vi "dI-dV(V) at various H_MFLI_MF-MD_K3636B_measureR_PK_V4.0_withaveraging.vi"() -> ()   [LabVIEW 2016]
uses:
  <instrlib>/Zurich Instruments LabOne/Public/Data/ziTypeDemodSampleSingle.ctl
  <instrlib>/Keithley 2600 Series/Public/Configure/Source/Configure Source (Limit).vi
  <instrlib>/Keithley 2600 Series/Public/Configure/Source/Configure Source (Range).vi
  <instrlib>/Zurich Instruments LabOne/Public/Configure/ziSetValueDouble.vi
  <instrlib>/Zurich Instruments LabOne/Public/Configure/ziGetValueDemodSampleEx.vi
  <instrlib>/Zurich Instruments LabOne/Zurich Instruments LabOne.lvlib
  <instrlib>/Keithley 2600 Series/Keithley 2600 Series.lvlib
panel:
  in  "MFLI autorange":bool
  in  "MFLI averaging":i32=100
  in  "Resistance used for DC (ohm)":dbl=20000000.0 format="%#_13g"
  in  "DC Current Limit (A)":dbl=0.001 format="%#_13g"
  in  "Keithley 2636B (channelA)":refnum<visa-resource-name>="GPIB0::26::INSTR"
  in  "Field ramp rate (T/min)":string="0.05"
  in  "Step 2":dbl[](array[numeric])=[0.01] min=-3000.0 max=3000.0 format="%.1e"
  in  "To 2":dbl[](array[numeric])=[1.0] min=-3000.0 max=3000.0 format="%.1e"
  in  "From 2":dbl[](array[numeric])=[1.0] min=-3000.0 max=3000.0 format="%.1e"
  in  "Magnet IP Address":string="169.254.239.127"
  in  "Magnetic field stabilization time (s)":dbl=10.0 format="%#_13g"
  out "Magnetic Field (T)":dbl=-9.479e-06 format="%#_13g"
  in  "DC Voltage averaging":dbl=20.0 format="%#_13g"
  out "Demod Sample Out 2":T1={"Timestamps (ticks)"=130270697085950, "X (Vrms)"=2.9261878078642585e-10, "Y (Vrms)"=-9.326090743141773e-11, "Osc Phase (deg)"=2.705175119436328, "Freq (Hz)"=137.91900016713043, "DIO"=0, "AuxIn0 (V)"=-1.5994189965713304, "AuxIn1 (V)"=0.0, "Trigger"=768}
  out "Demod Sample Out":T1={"Timestamps (ticks)"=130270395958270, "X (Vrms)"=1.8633428954504745e-05, "Y (Vrms)"=-1.3912734080062926e-05, "Osc Phase (deg)"=1.8681968520462253, "Freq (Hz)"=137.91900016713043, "DIO"=0, "AuxIn0 (V)"=-1.599753673071973, "AuxIn1 (V)"=0.0003336581285111606, "Trigger"=768}
  out "Vset (V)":dbl=-1.5999999999999879
  in  "stop":bool
  out "Time(s)":dbl=17491.89
  in  "Delay (s)":dbl=6.0
  out "dI/dV (S)":dbl=1.3195690059568667e-05
  out "dV (V)":dbl=2.3236791935984393e-05
  out "dI (A)":dbl=3.066255043659346e-10
  in  "MFLI Address":string="DEV4382"
  out "DC Voltage (V)":dbl=0.0024357376114999994
  in  "Folder":path=path "D:/Pranava/Data/STS/MA2087"
  out "dI/dV vs DC Bias (V)":cluster{dbl, "Field Reading":dbl}[](graph)=[{-0.0016267571685000004, "Field Reading"=1.2499190504022442e-05}, {-0.0016293047665, "Field Reading"=1.343983352593105e-05}, {-0.0016220483485, "Field Reading"=1.3498901551089376e-05}, {-0.0016165598575000003, "Field Reading"=1.3388711055940132e-05}, {-0.001611980558, "Field Reading"=1.3461634755634268e-05}, {-0.0016065861309999998, "Field Reading"=1.341362700532847e-05}, {-0.001602110838, "Field Reading"=1.3469326656062633e-05}, {-0.001603791602, "Field Reading"=1.3450198778996813e-05}, {-0.0016051868515, "Field Reading"=1.3453781776488028e-05}, {-0.0015975631075, "Field Reading"=1.3419416925134238e-05}, {-0.0015943920469999998, "Field Reading"=1.3462487063099248e-05}, {-0.001587995701, "Field Reading"=1.3450573702072532e-05}, {-0.0015837433415, "Field Reading"=1.3428263446816707e-05}, {-0.0015828466714999999, "Field Reading"=1.3393928336058793e-05}, {-0.0015733770785, "Field Reading"=1.3409612424077186e-05}, {-0.0015723401285000001, "Field Reading"=1.3483281690764093e-05}, {-0.001573338908, "Field Reading"=1.3468924481084309e-05}, {-0.0015673728475, "Field Reading"=1.3484666473714511e-05}, {-0.0015648761185, "Field Reading"=1.3459017041334516e-05}, {-0.0015634323450000002, "Field Reading"=1.3444091577240615e-05}, {-0.0015604055610000003, "Field Reading"=1.346636342471481e-05}, {-0.0015566468755, "Field Reading"=1.3440322960534301e-05}, {-0.0015575937835, "Field Reading"=1.3469711736300209e-05}, {-0.001552576611, "Field Reading"=1.3488882189349033e-05}, {-0.0015498932484999998, "Field Reading"=1.353533220023797e-05}, {-0.00154556704, "Field Reading"=1.3484237808051385e-05}, {-0.0015367533970000002, "Field Reading"=1.3408673038652877e-05}, {-0.0015292438589999996, "Field Reading"=1.3347996439904072e-05}, {-0.0015202704415000002, "Field Reading"=1.3380685506463923e-05}, {-0.0015157290055000001, "Field Reading"=1.3353547371126122e-05}, {-0.001518163067, "Field Reading"=1.3343450621350141e-05}, {-0.001513959626, "Field Reading"=1.3409316825027622e-05}, {-0.0015079468985, "Field Reading"=1.3565802247876391e-05}, {-0.00150523147, "Field Reading"=1.3366072109737657e-05}, {-0.0015025157965, "Field Reading"=1.3503176669159866e-05}, {-0.0015006006585000001, "Field Reading"=1.3475950682446334e-05}, {-0.0014965097129999998, "Field Reading"=1.343269307655852e-05}, {-0.0014928501455, "Field Reading"=1.3481127330206819e-05}, {-0.0014863147765, "Field Reading"=1.349537528914492e-05}, {-0.0014858813695000001, "Field Reading"=1.3464024342252269e-05}, {-0.0014759853594999998, "Field Reading"=1.3532450573952814e-05}, {-0.0014792820840000003, "Field Reading"=1.3467630784037758e-05}, {-0.0014737221895000003, "Field Reading"=1.3493114600583547e-05}, {-0.0014732275255000002, "Field Reading"=1.341814309027668e-05}, {-0.0014720142794999998, "Field Reading"=1.3430107894144245e-05}, {-0.0014674228615000002, "Field Reading"=1.3458062901131014e-05}, {-0.0014639780044999999, "Field Reading"=1.337799175960371e-05}, {-0.0014586194074999999, "Field Reading"=1.3432931895040972e-05}, {-0.0014546810515000002, "Field Reading"=1.3377936281541803e-05}, {-0.0014555862725000002, "Field Reading"=1.3440225961101887e-05}, {-0.0014500533295, "Field Reading"=1.3316922206414297e-05}, {-0.0014419232575, "Field Reading"=1.333479852156618e-05}, {-0.001439833057, "Field Reading"=1.335961205669311e-05}, {-0.001438517271, "Field Reading"=1.3276100719086655e-05}, {-0.001434182186, "Field Reading"=1.3414999580139993e-05}, {-0.0014277051765000004, "Field Reading"=1.3313685209980852e-05}, {-0.00142267889, "Field Reading"=1.3448885663949112e-05}, {-0.0014155909575, "Field Reading"=1.339123183517665e-05}, {-0.0014156524565, "Field Reading"=1.3297227349395088e-05}, {-0.0014124035680000001, "Field Reading"=1.3293565095925792e-05}, {-0.0014109490645, "Field Reading"=1.3394356468614784e-05}, {-0.001402366442, "Field Reading"=1.3391601134549928e-05}, {-0.001403825126, "Field Reading"=1.3292560889770096e-05}, {-0.0013966000125000002, "Field Reading"=1.3271969364171561e-05}, {-0.001394491805, "Field Reading"=1.3266411947286085e-05}, {-0.0013886783535, "Field Reading"=1.3363185326936124e-05}, {-0.0013879851079999998, "Field Reading"=1.3296944610611628e-05}, {-0.0013861102605, "Field Reading"=1.3375920541979456e-05}, {-0.001376159754, "Field Reading"=1.3268301330598542e-05}, {-0.0013715085824999999, "Field Reading"=1.3152900070607564e-05}, {-0.0013698944995, "Field Reading"=1.314215168062357e-05}, {-0.001366914667, "Field Reading"=1.3243900076650863e-05}, {-0.0013582629245000003, "Field Reading"=1.3197203437224588e-05}, {-0.0013513427565, "Field Reading"=1.3298167481611889e-05}, {-0.001352901842, "Field Reading"=1.3191445816026105e-05}, {-0.0013482640735, "Field Reading"=1.3131854012322067e-05}, {-0.0013431525900000003, "Field Reading"=1.319622184301407e-05}, {-0.0013453806239999999, "Field Reading"=1.3236450043175786e-05}, {-0.001338256563, "Field Reading"=1.3067235288946016e-05}, {-0.0013330496975, "Field Reading"=1.3278259509809853e-05}, {-0.001334601536, "Field Reading"=1.3161782791668972e-05}, {-0.0013293076895000001, "Field Reading"=1.3153363931625601e-05}, {-0.001328445928, "Field Reading"=1.3266280146530614e-05}, {-0.001323545566, "Field Reading"=1.3230633385568305e-05}, {-0.0013212523805, "Field Reading"=1.3153530500532615e-05}, {-0.001313054419, "Field Reading"=1.306718664169635e-05}, {-0.00131050229, "Field Reading"=1.3035829727727256e-05}, {-0.0013093692279999999, "Field Reading"=1.301171160959137e-05}, {-0.001300491978, "Field Reading"=1.3025217563977052e-05}, {-0.001291491248, "Field Reading"=1.2927163061100772e-05}, {-0.0012919785895, "Field Reading"=1.2950635606816967e-05}, {-0.0012839753905000003, "Field Reading"=1.295778636070639e-05}, {-0.001286123235, "Field Reading"=1.3035587121306979e-05}, {-0.001282255743, "Field Reading"=1.29379216298443e-05}, {-0.0012749608365, "Field Reading"=1.291957727591729e-05}, {-0.0012758108629999999, "Field Reading"=1.282723994321026e-05}, {-0.0012722698105000001, "Field Reading"=1.2806403042037306e-05}, {-0.001265646766, "Field Reading"=1.2866015068675188e-05}, {-0.0012694931415, "Field Reading"=1.2843347976402634e-05}, {-0.0012635237225, "Field Reading"=1.2985607427098843e-05}, {-0.0012617351054999997, "Field Reading"=1.3006933428484992e-05}, {-0.0012597806045, "Field Reading"=1.2885230079994883e-05}, {-0.0012488438765, "Field Reading"=1.2793535568477117e-05}, {-0.001242964541, "Field Reading"=1.2779432928316403e-05}, {-0.0012412559555, "Field Reading"=1.275312692545066e-05}, {-0.001240000649, "Field Reading"=1.2823591948584074e-05}, {-0.0012338296425, "Field Reading"=1.2753142420891901e-05}, {-0.0012334313899999999, "Field Reading"=1.260784282033363e-05}, {-0.0012307593545000002, "Field Reading"=1.2678998567641228e-05}, {-0.0012226835155000001, "Field Reading"=1.2531960406984556e-05}, {-0.0012170625415000003, "Field Reading"=1.2534788440635036e-05}, {-0.001215300631, "Field Reading"=1.2713738859126119e-05}, {-0.001214893501, "Field Reading"=1.2578666495750338e-05}, {-0.0012074607665, "Field Reading"=1.2623503148142356e-05}, {-0.0012017656785, "Field Reading"=1.2643045434630556e-05}, {-0.0011959136775, "Field Reading"=1.2531358907979804e-05}, {-0.001192863882, "Field Reading"=1.2682876125580679e-05}, {-0.001185345928, "Field Reading"=1.250172466195837e-05}, {-0.0011869023915000003, "Field Reading"=1.2401388355506459e-05}, {-0.001178852282, "Field Reading"=1.2735540228021439e-05}, {-0.0011705313045, "Field Reading"=1.2529360874641979e-05}, {-0.0011713601725000002, "Field Reading"=1.2406007363184931e-05}, {-0.001167284147, "Field Reading"=1.2562327760527226e-05}, {-0.0011657835375, "Field Reading"=1.2423839516376826e-05}, {-0.0011559746239999998, "Field Reading"=1.2409473414314111e-05}, {-0.0011557333085, "Field Reading"=1.223456105451975e-05}, {-0.00115341717, "Field Reading"=1.2267935976857073e-05}, {-0.0011506243345, "Field Reading"=1.2297468335684481e-05}, {-0.0011466437965, "Field Reading"=1.22625559418881e-05}, {-0.0011433223675, "Field Reading"=1.2313433576999384e-05}, {-0.0011387137115000002, "Field Reading"=1.2328609684580187e-05}, {-0.0011302218045, "Field Reading"=1.2448800178300881e-05}, {-0.001129965479, "Field Reading"=1.232422449512467e-05}, {-0.0011284153780000002, "Field Reading"=1.2457335401073954e-05}, {-0.0011258634070000005, "Field Reading"=1.2355751327365883e-05}, {-0.0011245481575, "Field Reading"=1.2398223740363219e-05}, {-0.0011186379170000003, "Field Reading"=1.2415162887415758e-05}, {-0.0011108317330000002, "Field Reading"=1.2234482045139758e-05}, {-0.0011040601549999998, "Field Reading"=1.239759514396126e-05}, {-0.0011008555040000001, "Field Reading"=1.2226625548810628e-05}, {-0.0010996387755, "Field Reading"=1.24008038522401e-05}, {-0.0010949081429999998, "Field Reading"=1.2406931342607784e-05}, {-0.0010871893910000003, "Field Reading"=1.2399554728236148e-05}, {-0.0010826407099999997, "Field Reading"=1.2455019484340595e-05}, {-0.0010847022115000001, "Field Reading"=1.2270122360570838e-05}, {-0.0010775761939999999, "Field Reading"=1.2426303312988743e-05}, {-0.0010693830505, "Field Reading"=1.2396176722109925e-05}, {-0.001068418253, "Field Reading"=1.2538655899985897e-05}, {-0.00105998586, "Field Reading"=1.2487974289067488e-05}, {-0.0010643841195, "Field Reading"=1.2022324173514663e-05}, {-0.0010465984804999997, "Field Reading"=1.237960545786543e-05}, {-0.001049693313, "Field Reading"=1.2357609137854957e-05}, {-0.0010453385914999998, "Field Reading"=1.2367705453586559e-05}, {-0.0010451289005000003, "Field Reading"=1.2179586177836105e-05}, {-0.0010427076885, "Field Reading"=1.2406396422746374e-05}, {-0.0010393730425000002, "Field Reading"=1.2264589264046061e-05}, {-0.001036272662, "Field Reading"=1.2232043251921527e-05}, {-0.0010331114714999998, "Field Reading"=1.2312089503579812e-05}, {-0.001024187028, "Field Reading"=1.2095593137600798e-05}, {-0.0010133286864999998, "Field Reading"=1.2022769275325186e-05}, {-0.0010093586194999998, "Field Reading"=1.2060485639315642e-05}, {-0.0010053248034999998, "Field Reading"=1.2176127116548629e-05}, {-0.00100089302075, "Field Reading"=1.212989507867769e-05}, {-0.0010046273665, "Field Reading"=1.2295865474738427e-05}, {-0.0009939405372999999, "Field Reading"=1.2570875611363628e-05}, {-0.00099936032935, "Field Reading"=1.2339198030666035e-05}, {-0.0009957504967, "Field Reading"=1.2451645025299093e-05}, {-0.00099513790295, "Field Reading"=1.2429995930400668e-05}, {-0.0009892875253999997, "Field Reading"=1.2072941232791506e-05}, {-0.0009848081800499999, "Field Reading"=1.2407152113702453e-05}, {-0.0009732798254999999, "Field Reading"=1.218132797601983e-05}, {-0.0009750383683499999, "Field Reading"=1.2502296174369174e-05}, {-0.00096801555695, "Field Reading"=1.2512782780469714e-05}, {-0.0009586896478999999, "Field Reading"=1.2515653591642282e-05}, {-0.00095599140395, "Field Reading"=1.2701841718895004e-05}, {-0.0009469954047, "Field Reading"=1.2304357333315858e-05}, {-0.0009383506428499999, "Field Reading"=1.2527858429029136e-05}, {-0.0009506185269000002, "Field Reading"=1.251948246858577e-05}, {-0.0009423335367000001, "Field Reading"=1.2454187258315746e-05}, {-0.0009380061563000001, "Field Reading"=1.2526322985323484e-05}, {-0.0009346829234999999, "Field Reading"=1.2468571394213803e-05}, {-0.0009271064448, "Field Reading"=1.2426604812429966e-05}, {-0.0009246051758, "Field Reading"=1.2504039467836049e-05}, {-0.0009237163829, "Field Reading"=1.2294098443501799e-05}, {-0.0009103104425499999, "Field Reading"=1.2548488043340115e-05}, {-0.0009141973994499999, "Field Reading"=1.2489954120047864e-05}, {-0.000919591549, "Field Reading"=1.2581967965222267e-05}, {-0.00091889418695, "Field Reading"=1.247930732400147e-05}, {-0.0009182332053500001, "Field Reading"=1.2549019013105507e-05}, {-0.0009119631786, "Field Reading"=1.254109078709283e-05}, {-0.00089912744415, "Field Reading"=1.2474940196701819e-05}, {-0.0008949993057000002, "Field Reading"=1.244505718344912e-05}, {-0.0008986060558, "Field Reading"=1.2436100406488695e-05}, {-0.0008897023131500001, "Field Reading"=1.2418263396906603e-05}, {-0.0008868790153500001, "Field Reading"=1.2428314253397502e-05}, {-0.0008768181397999999, "Field Reading"=1.2397124256484224e-05}, {-0.0008781432503, "Field Reading"=1.233446239627332e-05}, {-0.0008741251891999999, "Field Reading"=1.2339730990548692e-05}, {-0.0008662386407999999, "Field Reading"=1.2227294495302266e-05}, {-0.0008678619242, "Field Reading"=1.2178172676674001e-05}, {-0.0008564524111499998, "Field Reading"=1.2233860976341125e-05}, {-0.00083974567855, "Field Reading"=1.2174364874032163e-05}, {-0.0008426196614999999, "Field Reading"=1.2257540004764894e-05}, {-0.0008287142725, "Field Reading"=1.2065103433716045e-05}, {-0.0008285863424500001, "Field Reading"=1.2116775912153701e-05}, {-0.000820229371, "Field Reading"=1.214768997760333e-05}, {-0.000822172316, "Field Reading"=1.2140588348133439e-05}, {-0.00082194337245, "Field Reading"=1.2139858179971849e-05}, {-0.0008118778887, "Field Reading"=1.2152501764415964e-05}, {-0.0008042533364499999, "Field Reading"=1.1882766947604923e-05}, {-0.0008026405663, "Field Reading"=1.2073019153381417e-05}, {-0.0007960038935, "Field Reading"=1.1902004253937457e-05}, {-0.00080488926195, "Field Reading"=1.1534705081303725e-05}, {-0.0008023366587, "Field Reading"=1.123719732701356e-05}, {-0.0007833058507499999, "Field Reading"=1.1632902527488437e-05}, {-0.00078671102195, "Field Reading"=1.131615683017924e-05}, {-0.00077775515695, "Field Reading"=1.1504988617025489e-05}, {-0.00077084718225, "Field Reading"=1.14072188099698e-05}, {-0.000776439994, "Field Reading"=1.1043024243742828e-05}, {-0.0007647683212999999, "Field Reading"=1.1175000385507341e-05}, {-0.0007594209098000001, "Field Reading"=1.1139586423921927e-05}, {-0.00074996749215, "Field Reading"=1.1188552966499615e-05}, {-0.00075291306535, "Field Reading"=1.0770977673566891e-05}, {-0.00074549524615, "Field Reading"=1.0472371123959774e-05}, {-0.0007382761747, "Field Reading"=1.0676076384895258e-05}, {-0.00072738705785, "Field Reading"=1.0534548773470084e-05}, {-0.00072718818345, "Field Reading"=1.0033742603309901e-05}, {-0.0007257406150000001, "Field Reading"=1.0377769310827928e-05}, {-0.0007293339481500001, "Field Reading"=9.676816919051474e-06}, {-0.0007200138870000001, "Field Reading"=1.004746538174568e-05}, {-0.0007210630551499999, "Field Reading"=9.996160415018607e-06}, {-0.0007101231828, "Field Reading"=9.608375757846664e-06}, {-0.0007038174618499998, "Field Reading"=9.50044097891251e-06}, {-0.00070430843845, "Field Reading"=8.82521828814676e-06}, {-0.0006929104951, "Field Reading"=9.454696488523498e-06}, {-0.0006913446232999999, "Field Reading"=9.289499148448469e-06}, {-0.00069024800695, "Field Reading"=9.130635070279278e-06}, {-0.0006807302884999999, "Field Reading"=9.096673590989997e-06}, {-0.0006792669673, "Field Reading"=8.49565367874043e-06}, {-0.000674452605, "Field Reading"=8.791205115279277e-06}, {-0.0006605729285, "Field Reading"=8.616817121441707e-06}, {-0.0006493090853, "Field Reading"=8.744676457155707e-06}, {-0.0006483776634499999, "Field Reading"=8.411296973813767e-06}, {-0.0006424423944, "Field Reading"=8.30373914602951e-06}, {-0.00063679734075, "Field Reading"=8.09202314921175e-06}, {-0.0006310896040000001, "Field Reading"=7.935849345344011e-06}, {-0.0006187690644499999, "Field Reading"=7.530790237740172e-06}, {-0.0006142028893000001, "Field Reading"=7.467608340252136e-06}, {-0.0006122917381, "Field Reading"=7.429799980591347e-06}, {-0.00061505084645, "Field Reading"=7.507165251511274e-06}, {-0.0006130190451, "Field Reading"=7.477394946019876e-06}, {-0.0006092872664999998, "Field Reading"=7.4258372173230625e-06}, {-0.0006031213349000002, "Field Reading"=7.4007089463613716e-06}, {-0.0006068473796, "Field Reading"=7.363999614409341e-06}, {-0.000604482843, "Field Reading"=7.366692963412701e-06}, {-0.00060414160125, "Field Reading"=7.261092980188499e-06}, {-0.00060161189375, "Field Reading"=7.281630396042405e-06}, {-0.00059784590675, "Field Reading"=7.225758460870731e-06}, {-0.0005940079190500001, "Field Reading"=7.182783149976042e-06}, {-0.000598190185, "Field Reading"=7.132064037092618e-06}, {-0.0005920240745999999, "Field Reading"=7.089484731224047e-06}, {-0.0005936306892500001, "Field Reading"=7.142132013004073e-06}, {-0.00059292213345, "Field Reading"=7.021237323437015e-06}, {-0.00059135095375, "Field Reading"=6.793521649406981e-06}, {-0.00058789150445, "Field Reading"=7.117471722678135e-06}, {-0.0005897780709000001, "Field Reading"=6.925060626043223e-06}, {-0.0005877515152000001, "Field Reading"=7.169593917133456e-06}, {-0.0005882961062499999, "Field Reading"=7.1993621566164956e-06}, {-0.00058389374695, "Field Reading"=7.037649996827289e-06}, {-0.0005847123011499999, "Field Reading"=7.004853215553733e-06}, {-0.0005821565985000001, "Field Reading"=6.8965992497318605e-06}, {-0.00058612064725, "Field Reading"=6.451724993383642e-06}, {-0.0005807514161500001, "Field Reading"=6.791779790929323e-06}, {-0.0005770917991, "Field Reading"=6.9588968654746615e-06}, {-0.00057855298155, "Field Reading"=6.958157791235923e-06}, {-0.00057632977, "Field Reading"=6.822310091235498e-06}, {-0.00057638115055, "Field Reading"=7.03150935849712e-06}, {-0.0005694365351, "Field Reading"=6.848675323451398e-06}, {-0.0005690659662000001, "Field Reading"=6.348174970532446e-06}, {-0.0005641797593499999, "Field Reading"=6.378410563958051e-06}, {-0.00056214516005, "Field Reading"=6.261470669755067e-06}, {-0.00056095056685, "Field Reading"=6.2300331488003166e-06}, {-0.0005570344877, "Field Reading"=6.400854061035116e-06}, {-0.0005629947741999999, "Field Reading"=6.792009077572689e-06}, {-0.0005542106954500001, "Field Reading"=6.1953475193640665e-06}, {-0.00055450542695, "Field Reading"=6.368717915946041e-06}, {-0.00055000143825, "Field Reading"=6.1864670760017e-06}, {-0.0005598454800500001, "Field Reading"=6.31406909991541e-06}, {-0.00055229546895, "Field Reading"=6.41567665304393e-06}, {-0.0005567040322500001, "Field Reading"=6.162794755444581e-06}, {-0.00054615285805, "Field Reading"=6.278328666959152e-06}, {-0.0005495413454999999, "Field Reading"=6.535889902281644e-06}, {-0.0005496769236499998, "Field Reading"=6.50073721453714e-06}, {-0.0005447196448, "Field Reading"=6.300461498783274e-06}, {-0.00054405822255, "Field Reading"=6.702438316182959e-06}, {-0.00054522012775, "Field Reading"=6.522767423368897e-06}, {-0.00053720520805, "Field Reading"=6.505264299623565e-06}, {-0.00054277560625, "Field Reading"=6.551983667008787e-06}, {-0.000534306824, "Field Reading"=6.464861283181965e-06}, {-0.0005359110011, "Field Reading"=6.341609127317412e-06}, {-0.0005378842795, "Field Reading"=6.370016617424471e-06}, {-0.00053220733345, "Field Reading"=6.358633782071331e-06}, {-0.0005276139735500001, "Field Reading"=6.3590352355736425e-06}, {-0.00052423204045, "Field Reading"=6.244795262050721e-06}, {-0.00052568735385, "Field Reading"=6.3656544722698926e-06}, {-0.0005240912060000001, "Field Reading"=6.312395796471366e-06}, {-0.0005273072979, "Field Reading"=6.3307942677345504e-06}, {-0.0005263190813000001, "Field Reading"=6.431091429181517e-06}, {-0.0005218657422, "Field Reading"=6.4584700959617285e-06}, {-0.0005165821614499999, "Field Reading"=6.381246483496023e-06}, {-0.0005130783106000001, "Field Reading"=6.350888812041252e-06}, {-0.0005105342153, "Field Reading"=6.34358118431752e-06}, {-0.00051102444825, "Field Reading"=6.271602197981918e-06}, {-0.0005087865189000001, "Field Reading"=6.412714891370413e-06}, {-0.0005103624543000001, "Field Reading"=6.392942265197317e-06}, {-0.0005062118599, "Field Reading"=6.4240878869400706e-06}, {-0.0005033966741500001, "Field Reading"=6.324446092834119e-06}, {-0.0005029397692999999, "Field Reading"=6.319472364993404e-06}, {-0.00050283090065, "Field Reading"=6.348941112831489e-06}, {-0.0005058405701499999, "Field Reading"=6.34094319302428e-06}, {-0.0005026964292999999, "Field Reading"=6.357204323057684e-06}, {-0.0005009095037500001, "Field Reading"=6.393755081406965e-06}, {-0.00049469632955, "Field Reading"=6.323200793223342e-06}, {-0.0004981279740999999, "Field Reading"=6.395367007019279e-06}, {-0.0004982724323500001, "Field Reading"=6.382035815464461e-06}, {-0.0004922362558, "Field Reading"=6.399911646318677e-06}, {-0.0004925611278500002, "Field Reading"=6.425248731302264e-06}, {-0.0004880180931499999, "Field Reading"=6.381892573147459e-06}, {-0.00048794501634999985, "Field Reading"=6.397234702091804e-06}, {-0.00048763981149999995, "Field Reading"=6.4101260754235526e-06}, {-0.00048267884644999994, "Field Reading"=6.4176274966381554e-06}, {-0.00047489886809999994, "Field Reading"=6.410506476510949e-06}, {-0.000472017602, "Field Reading"=6.406149278197199e-06}, {-0.00047454752534999996, "Field Reading"=6.434172488891919e-06}, {-0.00047850674865000003, "Field Reading"=6.460926732775075e-06}, {-0.00047843549325, "Field Reading"=6.460369593726035e-06}, {-0.00047903993434999994, "Field Reading"=6.543217810373611e-06}, {-0.00047349881965000004, "Field Reading"=6.475239774184411e-06}, {-0.0004740396457, "Field Reading"=6.456118391900139e-06}, {-0.00046971869225, "Field Reading"=6.5215079995270816e-06}, {-0.00046948385280000014, "Field Reading"=6.504040037231308e-06}, {-0.0004682857755, "Field Reading"=6.543077945122342e-06}, {-0.00046408979245000004, "Field Reading"=6.5569532654151625e-06}, {-0.0004678369874, "Field Reading"=6.509755580474492e-06}, {-0.00046764634865, "Field Reading"=6.564630011682037e-06}, {-0.0004668231169, "Field Reading"=6.579497702445634e-06}, {-0.00046441008514999996, "Field Reading"=6.579350067368638e-06}, {-0.00045738932385, "Field Reading"=6.672754541853891e-06}, {-0.00046233230790000007, "Field Reading"=6.646848361809121e-06}, {-0.00046401533655, "Field Reading"=6.647284914749344e-06}, {-0.0004573838583, "Field Reading"=6.643135354100359e-06}, {-0.00045558283854999995, "Field Reading"=6.707567976292288e-06}, {-0.0004458977102, "Field Reading"=6.7232426784355734e-06}, {-0.0004474432096, "Field Reading"=6.7747372082633595e-06}, {-0.0004453321657500001, "Field Reading"=6.787371582123838e-06}, {-0.00044470507725, "Field Reading"=6.830027579717506e-06}, {-0.00044548761405, "Field Reading"=6.856783686685118e-06}, {-0.0004474259934, "Field Reading"=6.771487748449478e-06}, {-0.0004446336348, "Field Reading"=6.829699993004862e-06}, {-0.00043687574165, "Field Reading"=6.906930682770715e-06}, {-0.00044126883650000005, "Field Reading"=6.775872705880396e-06}, {-0.00043802800954999987, "Field Reading"=6.801703069808951e-06}, {-0.00043858563210000007, "Field Reading"=6.787492487038415e-06}, {-0.0004356597395, "Field Reading"=6.906599833714602e-06}, {-0.00043092829495000004, "Field Reading"=7.0581726788019045e-06}, {-0.00042655147195, "Field Reading"=7.073170063820467e-06}, {-0.00043001205805, "Field Reading"=7.078483055696094e-06}, {-0.0004312922125, "Field Reading"=6.9117169228160235e-06}, {-0.00043052456884999993, "Field Reading"=6.950272124357718e-06}, {-0.00043010766104999994, "Field Reading"=7.032954001081137e-06}, {-0.00042734102690000005, "Field Reading"=6.982349159757663e-06}, {-0.0004239069480500001, "Field Reading"=6.9919914097777005e-06}, {-0.00042524036374999997, "Field Reading"=7.020189298550575e-06}, {-0.00043156011754999995, "Field Reading"=7.076642632296424e-06}, {-0.00042715297519999994, "Field Reading"=7.066236233115896e-06}, {-0.0004186479316, "Field Reading"=7.163115599392733e-06}, {-0.00041536434724999996, "Field Reading"=7.380892439560495e-06}, {-0.0004131149345000001, "Field Reading"=7.440972271186679e-06}, {-0.0004189563549, "Field Reading"=7.299538763321159e-06}, {-0.0004194009282500001, "Field Reading"=7.296277913012798e-06}, {-0.00041866060545, "Field Reading"=7.2622495426002635e-06}, {-0.00041365388355000003, "Field Reading"=7.260454883104575e-06}, {-0.00041438161699999994, "Field Reading"=7.294900456366183e-06}, {-0.00041219219255, "Field Reading"=7.305175418458287e-06}, {-0.0004132851208499999, "Field Reading"=7.274758893032781e-06}, {-0.0004105045459, "Field Reading"=7.298280624006913e-06}, {-0.00040969569465, "Field Reading"=7.342113366818655e-06}, {-0.00041067156875, "Field Reading"=7.386682730824256e-06}, {-0.00041137594874999996, "Field Reading"=7.394748816204072e-06}, {-0.00040986792535000003, "Field Reading"=7.418747016182462e-06}, {-0.00040415003255, "Field Reading"=7.503290731073102e-06}, {-0.00040549978755, "Field Reading"=7.5415442861903745e-06}, {-0.00039870969664999997, "Field Reading"=7.531249386235733e-06}, {-0.0003971851577, "Field Reading"=7.529644369399869e-06}, {-0.0003978213472, "Field Reading"=7.561749097048822e-06}, {-0.00040007185540000007, "Field Reading"=7.560137044704404e-06}, {-0.0003994220251, "Field Reading"=7.572984734830169e-06}, {-0.00039392529455, "Field Reading"=7.612319531344689e-06}, {-0.00039373372194999995, "Field Reading"=7.5973383115281384e-06}, {-0.00039226355145, "Field Reading"=7.72173548690546e-06}, {-0.00038828587340000004, "Field Reading"=7.852235680298321e-06}, {-0.00038698300425, "Field Reading"=7.841915060373217e-06}, {-0.00038667021055, "Field Reading"=7.840163045482861e-06}, {-0.0003822117375, "Field Reading"=7.885235150327136e-06}, {-0.0003777846756, "Field Reading"=7.8665315535847e-06}, {-0.0003761510863, "Field Reading"=7.842199128310843e-06}, {-0.00038040052425, "Field Reading"=7.917983703122608e-06}, {-0.00037604463869999997, "Field Reading"=7.929201302881441e-06}, {-0.00037606562759999994, "Field Reading"=7.900022479503202e-06}, {-0.00037312674575, "Field Reading"=7.897148441545767e-06}, {-0.0003752304105, "Field Reading"=7.968871544358153e-06}, {-0.00037971265935, "Field Reading"=8.035260921543662e-06}, {-0.00037442999985, "Field Reading"=8.004491783319515e-06}, {-0.00036828163960000006, "Field Reading"=8.045504296326132e-06}, {-0.00037103631005000004, "Field Reading"=8.031684488280136e-06}, {-0.0003704617713, "Field Reading"=8.135555434624158e-06}, {-0.00036746019310000003, "Field Reading"=8.181218688385326e-06}, {-0.00036643864434999997, "Field Reading"=8.117505798392926e-06}, {-0.00036547628895, "Field Reading"=8.194388535497674e-06}, {-0.0003644862809, "Field Reading"=8.129337463184387e-06}, {-0.00036567006105000003, "Field Reading"=8.123409993780417e-06}, {-0.00036820808259999994, "Field Reading"=8.079144338866577e-06}, {-0.0003693601304499999, "Field Reading"=8.182903278863496e-06}, {-0.00036751546295, "Field Reading"=8.186745458268257e-06}, {-0.00036839839184999996, "Field Reading"=8.171277569471231e-06}, {-0.00036140248015, "Field Reading"=8.165911663178433e-06}, {-0.00035908212725, "Field Reading"=8.296580150801212e-06}, {-0.00036057380724999996, "Field Reading"=8.180237413212517e-06}, {-0.000360656483, "Field Reading"=8.317984064260158e-06}, {-0.00035712477125000007, "Field Reading"=8.269041451300612e-06}, {-0.00035295078870000004, "Field Reading"=8.342918996307952e-06}, {-0.0003527069946, "Field Reading"=8.43699640626219e-06}, {-0.00035016069329999995, "Field Reading"=8.431029157642895e-06}, {-0.00035228532085000003, "Field Reading"=8.428806876729552e-06}, {-0.00035130559819999995, "Field Reading"=8.470623589987256e-06}, {-0.00034789776725, "Field Reading"=8.485770660484109e-06}, {-0.0003459226942, "Field Reading"=8.57467240380038e-06}, {-0.00034298782725, "Field Reading"=8.439862262657038e-06}, {-0.00034257298325000005, "Field Reading"=8.42040765457595e-06}, {-0.00034698661579999994, "Field Reading"=8.4132433736633e-06}, {-0.0003452512637, "Field Reading"=8.452215948675254e-06}, {-0.00034221470775, "Field Reading"=8.451875118368673e-06}, {-0.00034152220055, "Field Reading"=8.503401828755911e-06}, {-0.00034139717825, "Field Reading"=8.45504491950377e-06}, {-0.0003426610638, "Field Reading"=8.454731850061626e-06}, {-0.00033969001525, "Field Reading"=8.516243097363457e-06}, {-0.00033749485995, "Field Reading"=8.52040695934161e-06}, {-0.00033796018544999997, "Field Reading"=8.470074351000046e-06}, {-0.00033421099610000005, "Field Reading"=8.429381039810805e-06}, {-0.00033249144774999997, "Field Reading"=8.483892783076501e-06}, {-0.0003321798061, "Field Reading"=8.540764565622142e-06}, {-0.00032731269235, "Field Reading"=8.518749606552973e-06}, {-0.0003258160537, "Field Reading"=8.541617971045343e-06}, {-0.00032094227625000004, "Field Reading"=8.50726446077068e-06}, {-0.00032337393499999996, "Field Reading"=8.599982186631013e-06}, {-0.00031622440355, "Field Reading"=8.594097518864634e-06}, {-0.00031394453295, "Field Reading"=8.642190907561487e-06}, {-0.0003126196953, "Field Reading"=8.611204139292685e-06}, {-0.00031092731875, "Field Reading"=8.570922167609616e-06}, {-0.00031113745555, "Field Reading"=8.639412275063455e-06}, {-0.0003170082651000001, "Field Reading"=8.642601498905943e-06}, {-0.00031539928415, "Field Reading"=8.664640662791292e-06}, {-0.00031388043945, "Field Reading"=8.674153933745916e-06}, {-0.000312063405, "Field Reading"=8.681190482579656e-06}, {-0.00031397822165, "Field Reading"=8.622785335838662e-06}, {-0.0003098279338500001, "Field Reading"=8.658652750588886e-06}, {-0.00030971474885000007, "Field Reading"=8.62974193982224e-06}, {-0.00030778190044999996, "Field Reading"=8.688824457808184e-06}, {-0.00030806160849999994, "Field Reading"=8.707117448002158e-06}, {-0.000308639312, "Field Reading"=8.728329131110018e-06}, {-0.00030851778285, "Field Reading"=8.703292227605214e-06}, {-0.00030481103215000005, "Field Reading"=8.713950872572662e-06}, {-0.00030326751710000005, "Field Reading"=8.749334580294675e-06}, {-0.00029831044145, "Field Reading"=8.826461353074001e-06}, {-0.0002951900614, "Field Reading"=8.832828052582353e-06}, {-0.00029633771065, "Field Reading"=8.825251690470345e-06}, {-0.00029650410709999994, "Field Reading"=8.828961487477813e-06}, {-0.00029445616885, "Field Reading"=8.83815527915802e-06}, {-0.0002920261708, "Field Reading"=8.810706124839746e-06}, {-0.0002942481603500001, "Field Reading"=8.835467569138388e-06}, {-0.00029624758055, "Field Reading"=8.87212672787701e-06}, {-0.00029012604135, "Field Reading"=8.868554330137962e-06}, {-0.00029241337785, "Field Reading"=8.876134594846024e-06}, {-0.00028751735475000004, "Field Reading"=8.905922302552472e-06}, {-0.00029197494704999997, "Field Reading"=8.956938854321487e-06}, {-0.0002905404879, "Field Reading"=8.92004300889604e-06}, {-0.00028727119275, "Field Reading"=8.905269138187045e-06}, {-0.00028416392770000003, "Field Reading"=8.901317064172347e-06}, {-0.00028469630984999996, "Field Reading"=8.917208240689476e-06}, {-0.00028069842905, "Field Reading"=8.939538207996445e-06}, {-0.00028365025759999996, "Field Reading"=8.947268156394279e-06}, {-0.00028181174155, "Field Reading"=8.930092789559604e-06}, {-0.00028018209845, "Field Reading"=8.994196176297592e-06}, {-0.00028035463059999997, "Field Reading"=8.97671386371425e-06}, {-0.00028007555434999995, "Field Reading"=8.992829735439781e-06}, {-0.00028165055950000003, "Field Reading"=9.010103482939582e-06}, {-0.0002818198449, "Field Reading"=9.03573201948662e-06}, {-0.00027695776855, "Field Reading"=8.988708588452728e-06}, {-0.00027290522435, "Field Reading"=9.012338142187786e-06}, {-0.00027415493029999994, "Field Reading"=8.975830469345412e-06}, {-0.00027867530340000004, "Field Reading"=9.07409242274734e-06}, {-0.00027804220155, "Field Reading"=9.092480236995706e-06}, {-0.00027876582905000003, "Field Reading"=9.050862031133768e-06}, {-0.00027262430685, "Field Reading"=9.026789442364259e-06}, {-0.0002711804288, "Field Reading"=9.102530935914161e-06}, {-0.00027107232180000003, "Field Reading"=9.085823574781249e-06}, {-0.0002710472894, "Field Reading"=9.090749991874897e-06}, {-0.0002713672529, "Field Reading"=9.119570982152522e-06}, {-0.0002700028398, "Field Reading"=9.110452309854145e-06}, {-0.00026849136605, "Field Reading"=9.142880954030727e-06}, {-0.00026452950475, "Field Reading"=9.132430383382145e-06}, {-0.00026477639545000004, "Field Reading"=9.149319412753625e-06}, {-0.0002632882570500001, "Field Reading"=9.193253615538679e-06}, {-0.0002584906278, "Field Reading"=9.20454452658872e-06}, {-0.0002542380579, "Field Reading"=9.234667189014463e-06}, {-0.00025207493105, "Field Reading"=9.224236206177708e-06}, {-0.00025094732335, "Field Reading"=9.226313226953917e-06}, {-0.00025213711035, "Field Reading"=9.224641393273539e-06}, {-0.00025010687619999997, "Field Reading"=9.231969636450967e-06}, {-0.00024825372010000007, "Field Reading"=9.276432630864505e-06}, {-0.0002449619948, "Field Reading"=9.236150749245714e-06}, {-0.00024610099095, "Field Reading"=9.26246697283035e-06}, {-0.00024617457365, "Field Reading"=9.26276769297323e-06}, {-0.0002476271681, "Field Reading"=9.25967590597896e-06}, {-0.00024411954485, "Field Reading"=9.248996931807503e-06}, {-0.00024134129335, "Field Reading"=9.244251283883492e-06}, {-0.00024215462090000002, "Field Reading"=9.255840070350768e-06}, {-0.00023799151944999997, "Field Reading"=9.207430137152989e-06}, {-0.000243466289, "Field Reading"=9.177226091439831e-06}, {-0.00023932615135000002, "Field Reading"=9.187628169586353e-06}, {-0.00023556527210000008, "Field Reading"=9.17694969628356e-06}, {-0.0002364329548, "Field Reading"=9.222668220432728e-06}, {-0.00023408173255000001, "Field Reading"=9.241119639424134e-06}, {-0.00022868252090000007, "Field Reading"=9.167297450171014e-06}, {-0.00023043670005, "Field Reading"=9.158561225950368e-06}, {-0.00023036615475000006, "Field Reading"=9.108033630084853e-06}, {-0.00022943969205000003, "Field Reading"=9.10614626417229e-06}, {-0.00022689811785, "Field Reading"=9.072414804875704e-06}, {-0.00022690312525000005, "Field Reading"=9.069668772595963e-06}, {-0.00022950191234999998, "Field Reading"=9.080168492196367e-06}, {-0.00022680520910000002, "Field Reading"=9.048489092014522e-06}, {-0.00022237740155, "Field Reading"=8.953998414918463e-06}, {-0.00022449479689999998, "Field Reading"=8.943012712035921e-06}, {-0.0002259390296, "Field Reading"=8.902165272024735e-06}, {-0.0002247596057, "Field Reading"=8.829806945551352e-06}, {-0.00022329492655000002, "Field Reading"=8.796390381915911e-06}, {-0.00022196154975000004, "Field Reading"=8.695632437475198e-06}, {-0.0002202722261, "Field Reading"=8.67354457392291e-06}, {-0.00021900004014999995, "Field Reading"=8.586022677127473e-06}, {-0.00021841042069999997, "Field Reading"=8.517711788682228e-06}, {-0.0002192617544, "Field Reading"=8.469275920940975e-06}, {-0.00021618217674999998, "Field Reading"=8.407782351157063e-06}, {-0.00021648695950000002, "Field Reading"=8.40019403507054e-06}, {-0.00021225518655, "Field Reading"=8.378152960068131e-06}, {-0.00021070851015, "Field Reading"=8.20914304982398e-06}, {-0.00020675074105000005, "Field Reading"=8.132382787637307e-06}, {-0.00021101619075, "Field Reading"=8.051468048856455e-06}, {-0.00020820556365, "Field Reading"=7.979384176413048e-06}, {-0.00020550454335, "Field Reading"=7.917320415480876e-06}, {-0.00020525080129999996, "Field Reading"=7.821458826881498e-06}, {-0.00020482333835, "Field Reading"=7.730716134592994e-06}, {-0.00020338587755, "Field Reading"=7.52649513275565e-06}, {-0.0001997145949, "Field Reading"=7.495184539796538e-06}, {-0.00020153224269999994, "Field Reading"=7.437453391188783e-06}, {-0.0002018581807, "Field Reading"=7.238917675419438e-06}, {-0.00019718399255, "Field Reading"=7.0735019259360834e-06}, {-0.00019440910949999998, "Field Reading"=6.9231598352528615e-06}, {-0.00019236311389999997, "Field Reading"=6.78084291006387e-06}, {-0.00019218741629999997, "Field Reading"=6.654064538863958e-06}, {-0.00019274157575000002, "Field Reading"=6.583459052982115e-06}, {-0.0001886177745, "Field Reading"=6.44972326268537e-06}, {-0.00018765849304999997, "Field Reading"=6.272426771312183e-06}, {-0.00018745534180000003, "Field Reading"=6.149644336326817e-06}, {-0.0001840720801, "Field Reading"=5.989973883433464e-06}, {-0.0001823129922, "Field Reading"=5.8266257309747445e-06}, {-0.0001799855923, "Field Reading"=5.7468656344964e-06}, {-0.00017918058035000002, "Field Reading"=5.514170597795423e-06}, {-0.0001762393677, "Field Reading"=5.302993415358113e-06}, {-0.00017500609080000004, "Field Reading"=5.157445043642254e-06}, {-0.00016575431969999998, "Field Reading"=5.057186396822109e-06}, {-0.00017013088749999998, "Field Reading"=4.837690143214849e-06}, {-0.00016389061545, "Field Reading"=4.683232223957943e-06}, {-0.00016383600175, "Field Reading"=4.515961124348759e-06}, {-0.00016330939689999997, "Field Reading"=4.284672212601775e-06}, {-0.0001567752275, "Field Reading"=4.1535477519381926e-06}, {-0.0001593526425, "Field Reading"=3.885568004005577e-06}, {-0.00015647927159999998, "Field Reading"=3.6759503115456187e-06}, {-0.00015341407444999998, "Field Reading"=3.5637640417285483e-06}, {-0.0001511484693, "Field Reading"=3.469285865323771e-06}, {-0.00014996206355, "Field Reading"=3.2250641902237846e-06}, {-0.00015501180155, "Field Reading"=3.099635633321275e-06}, {-0.00015195596395, "Field Reading"=2.943985354060433e-06}, {-0.00014620904955, "Field Reading"=2.7461367253135745e-06}, {-0.0001406028873, "Field Reading"=2.4777211837384678e-06}, {-0.0001365053755, "Field Reading"=2.2401381152299947e-06}, {-0.00013696148585, "Field Reading"=2.2169434938600603e-06}, {-0.00013117720555000002, "Field Reading"=1.920089955640667e-06}, {-0.00012309311445, "Field Reading"=1.6963298891703644e-06}, {-0.00011506420559999999, "Field Reading"=1.6036232732303053e-06}, {-0.00010885863545, "Field Reading"=1.4911623569271934e-06}, {-0.00010859234445000001, "Field Reading"=1.3568335337515127e-06}, {-9.743801383500001e-05, "Field Reading"=1.1615555396584243e-06}, {-9.1135923385e-05, "Field Reading"=1.0057022815055216e-06}, {-8.314956718999999e-05, "Field Reading"=8.467831454022928e-07}, {-7.195333897499999e-05, "Field Reading"=7.239202249151924e-07}, {-5.6697478795e-05, "Field Reading"=5.658617724441297e-07}, {-3.776427648999999e-05, "Field Reading"=4.6449750608729116e-07}, {-2.393483787e-05, "Field Reading"=3.7462582593470653e-07}, {-1.1536860103500001e-05, "Field Reading"=2.823566255515183e-07}, {2.838831519e-05, "Field Reading"=1.924612671957555e-07}, {7.6288298175e-05, "Field Reading"=1.1588526508005153e-07}, {0.0002025768314, "Field Reading"=1.8555721385175304e-08}, {0.0004762918990499999, "Field Reading"=2.5337248384286484e-08}, {0.0006709073683, "Field Reading"=8.662156050408576e-08}, {0.0007349988097, "Field Reading"=1.9725817711875567e-07}, {0.00076453909985, "Field Reading"=2.9295699190872743e-07}, {0.00078880062965, "Field Reading"=3.8519797026104865e-07}, {0.00080942795205, "Field Reading"=4.5869691557925045e-07}, {0.0008324251998500001, "Field Reading"=5.881502155601284e-07}, {0.0008439205607000001, "Field Reading"=7.404156793632427e-07}, {0.000848416117, "Field Reading"=9.06637309790864e-07}, {0.0008600555814000001, "Field Reading"=1.0130327524666915e-06}, {0.0008655675055999999, "Field Reading"=1.200032798054732e-06}, {0.0008678505505, "Field Reading"=1.3365257637198908e-06}, {0.0008757079878999999, "Field Reading"=1.5396933405698614e-06}, {0.0008817874388, "Field Reading"=1.6858883337799816e-06}, {0.0008898672299000002, "Field Reading"=1.868390759658339e-06}, {0.0008869096864499999, "Field Reading"=2.0364806486958376e-06}, {0.00088928925715, "Field Reading"=2.158136434046408e-06}, {0.00089503293485, "Field Reading"=2.395896854418827e-06}, {0.0009026049111500002, "Field Reading"=2.5573896059995884e-06}, {0.0009047032375499999, "Field Reading"=2.7522247762329643e-06}, {0.00090723065655, "Field Reading"=2.8938001693180717e-06}, {0.0009106404856499998, "Field Reading"=3.100134766058298e-06}, {0.0009137064031, "Field Reading"=3.2732276680523986e-06}, {0.0009213144410500001, "Field Reading"=3.370692929301835e-06}, {0.0009265759572500001, "Field Reading"=3.648823970439872e-06}, {0.0009217140466000001, "Field Reading"=3.793638820862184e-06}, {0.0009249784430499999, "Field Reading"=3.906147455462879e-06}, {0.0009254545098499999, "Field Reading"=4.1193634279466376e-06}, {0.0009304776045999999, "Field Reading"=4.286388453463172e-06}, {0.0009349188306000001, "Field Reading"=4.431130350347026e-06}, {0.0009399908263500002, "Field Reading"=4.562914522501731e-06}, {0.00094190377475, "Field Reading"=4.757027396535464e-06}, {0.0009465729132499999, "Field Reading"=4.888797741140083e-06}, {0.0009482012894, "Field Reading"=5.005568924171559e-06}, {0.0009471116324999999, "Field Reading"=5.144862643556753e-06}, {0.0009493125639, "Field Reading"=5.326421921939137e-06}, {0.0009519107324999999, "Field Reading"=5.424727748922771e-06}, {0.0009526514079500001, "Field Reading"=5.567844817903921e-06}, {0.00095669410805, "Field Reading"=5.653561079434558e-06}, {0.0009592396140000001, "Field Reading"=5.759461167637162e-06}, {0.0009581738822499998, "Field Reading"=5.9017985100211325e-06}, {0.0009629995314500001, "Field Reading"=6.015555683664982e-06}, {0.0009634269349500001, "Field Reading"=6.109091293063464e-06}, {0.0009638469428000002, "Field Reading"=6.169325375983161e-06}, {0.0009672600367999998, "Field Reading"=6.27096897792405e-06}, {0.0009714622430500001, "Field Reading"=6.3279137208837415e-06}, {0.000969406538, "Field Reading"=6.417517729637328e-06}, {0.00096806096415, "Field Reading"=6.51270036706873e-06}, {0.0009729091635000001, "Field Reading"=6.560168422439599e-06}, {0.0009713268937000001, "Field Reading"=6.620875251523027e-06}, {0.0009801303540499999, "Field Reading"=6.632621387546809e-06}, {0.0009802664602499998, "Field Reading"=6.713500885436769e-06}, {0.00097650758105, "Field Reading"=6.790044811584047e-06}, {0.0009775937964499998, "Field Reading"=6.8802061377682245e-06}, {0.00098226362805, "Field Reading"=6.900949448809808e-06}, {0.0009825031792499998, "Field Reading"=6.912481104060984e-06}, {0.0009831856460499999, "Field Reading"=6.888286810064999e-06}, {0.00098630398055, "Field Reading"=7.001121469814767e-06}, {0.0009919814813499999, "Field Reading"=7.0346064067925705e-06}, {0.00099628020535, "Field Reading"=7.057637428125096e-06}, {0.0010058769525, "Field Reading"=6.938435920576142e-06}, {0.0010163268349999998, "Field Reading"=6.849355597651672e-06}, {0.0010222887739999996, "Field Reading"=6.6278220630651525e-06}, {0.0010325292675, "Field Reading"=6.410026424822375e-06}, {0.0010406998, "Field Reading"=6.179822425214637e-06}, {0.0010472690229999999, "Field Reading"=5.977475271201429e-06}, {0.0010578505685, "Field Reading"=5.767966464215794e-06}, {0.0010657538055, "Field Reading"=5.5744713762265145e-06}, {0.0010714282789999999, "Field Reading"=5.322000420642119e-06}, {0.0010850249275, "Field Reading"=5.163347077542497e-06}, {0.0010926668075, "Field Reading"=4.976190523405071e-06}, {0.0011021957994999999, "Field Reading"=4.8281586235485565e-06}, {0.0011135380554999998, "Field Reading"=4.651081376155409e-06}, {0.0011270981674999998, "Field Reading"=4.563774407289007e-06}, {0.001136447252, "Field Reading"=4.468847017765011e-06}, {0.0011480480269999997, "Field Reading"=4.391198727722254e-06}, {0.0011602018685, "Field Reading"=4.334502912453376e-06}, {0.001173553335, "Field Reading"=4.268338399285161e-06}, {0.001185902166, "Field Reading"=4.2568472870556015e-06}, {0.0011991425465, "Field Reading"=4.218434030199776e-06}, {0.0012091100315000003, "Field Reading"=4.268602664540743e-06}, {0.0012196680255, "Field Reading"=4.2899418992222325e-06}, {0.0012297030205, "Field Reading"=4.369457451303169e-06}, {0.0012388505315, "Field Reading"=4.441880164740922e-06}, {0.001249947689, "Field Reading"=4.4976832611244295e-06}, {0.001259238686, "Field Reading"=4.682489179096483e-06}, {0.00127322495, "Field Reading"=4.772523824866306e-06}, {0.0012854579755, "Field Reading"=4.884926873492575e-06}, {0.0012942291745, "Field Reading"=4.983456010900706e-06}, {0.0012994435505000001, "Field Reading"=5.054190627581887e-06}, {0.001312025137, "Field Reading"=5.214714608352841e-06}, {0.0013188658054999998, "Field Reading"=5.185168484164302e-06}, {0.0013275724865000002, "Field Reading"=5.67289124340211e-06}, {0.0013389099949999998, "Field Reading"=5.730280029944138e-06}, {0.0013500877154999998, "Field Reading"=6.0890216252628145e-06}, {0.0013542734090000001, "Field Reading"=6.182944346777105e-06}, {0.0013624477685, "Field Reading"=6.258520329644863e-06}, {0.001371577464, "Field Reading"=6.541734950792698e-06}, {0.0013790151594999997, "Field Reading"=6.631959653303689e-06}, {0.0013870042765, "Field Reading"=6.785583521274233e-06}, {0.001394643245, "Field Reading"=6.771977329071211e-06}, {0.0013972065014999997, "Field Reading"=7.149734087780881e-06}, {0.0014057592805, "Field Reading"=7.295957122297294e-06}, {0.001408718353, "Field Reading"=7.497081544634262e-06}, {0.0014134534185, "Field Reading"=7.601625757117305e-06}, {0.0014211648615000002, "Field Reading"=7.545209696171624e-06}, {0.0014284192595000003, "Field Reading"=7.970695752287871e-06}, {0.0014357070355000001, "Field Reading"=7.906823217269699e-06}, {0.001442501744, "Field Reading"=7.960579579413913e-06}, {0.0014504179934999998, "Field Reading"=8.027664347223766e-06}, {0.0014533098609999999, "Field Reading"=8.313841580253358e-06}, {0.0014594672965, "Field Reading"=8.714627129528964e-06}, {0.0014677408279999999, "Field Reading"=8.392342494718513e-06}, {0.0014770621025000001, "Field Reading"=8.79541225629204e-06}, {0.0014837886745000001, "Field Reading"=8.840868757866375e-06}, {0.001488784217, "Field Reading"=9.050704644171554e-06}, {0.0014905906935, "Field Reading"=9.071075608012616e-06}, {0.0014999342425000002, "Field Reading"=9.163298077949285e-06}, {0.001508746947, "Field Reading"=9.126491128277866e-06}, {0.0015122893219999998, "Field Reading"=9.313948216527783e-06}, {0.0015180174789999998, "Field Reading"=9.544719584375942e-06}, {0.0015254218205, "Field Reading"=9.549548062539699e-06}, {0.0015281683765, "Field Reading"=9.799730522262928e-06}, {0.0015364120544999998, "Field Reading"=9.954500769772188e-06}, {0.0015421077890000001, "Field Reading"=9.999625907788466e-06}, {0.001541882135, "Field Reading"=1.0023957336835575e-05}, {0.0015569535799999999, "Field Reading"=1.0167564259440324e-05}, {0.0015598654985, "Field Reading"=1.0289943492441287e-05}, {0.0015590741565000002, "Field Reading"=1.0293154857689109e-05}, {0.0015611509575, "Field Reading"=1.0355781328564268e-05}, {0.001562708603, "Field Reading"=1.0432942044567697e-05}, {0.0015645545865, "Field Reading"=1.064812242682252e-05}, {0.0015647676395000002, "Field Reading"=1.0754160115055755e-05}, {0.0015746865240000001, "Field Reading"=1.0858443434886712e-05}, {0.0015760858455, "Field Reading"=1.091096223730189e-05}, {0.0015868030030000001, "Field Reading"=1.0968019155545074e-05}, {0.00158850574, "Field Reading"=1.101570732723819e-05}, {0.0015939327765, "Field Reading"=1.1116901079167024e-05}, {0.0016022500379999998, "Field Reading"=1.1206175880780007e-05}, {0.001603253728, "Field Reading"=1.1335098725304137e-05}, {0.0016055945789999998, "Field Reading"=1.1376489680362105e-05}, {0.0016126402615, "Field Reading"=1.1378057846391138e-05}, {0.0016123194579999995, "Field Reading"=1.1454274777949144e-05}, {0.0016200421225, "Field Reading"=1.1601453017406494e-05}, {0.0016308237905, "Field Reading"=1.1613246377602089e-05}, {0.0016269435550000002, "Field Reading"=1.1716814083853476e-05}, {0.0016327594105, "Field Reading"=1.1877591211581334e-05}, {0.0016424699590000002, "Field Reading"=1.197196659901818e-05}, {0.0016450608980000004, "Field Reading"=1.1960404001304426e-05}, {0.0016478802025000003, "Field Reading"=1.2009216866206365e-05}, {0.0016480433670000003, "Field Reading"=1.203610138725264e-05}, {0.0016550793424999998, "Field Reading"=1.2225826792218882e-05}, {0.0016654934139999997, "Field Reading"=1.2208763507207508e-05}, {0.0016682392635000002, "Field Reading"=1.2336692553441846e-05}, {0.0016657489645, "Field Reading"=1.2345866130415325e-05}, {0.0016684598865, "Field Reading"=1.2370470194520026e-05}, {0.0016740523635000002, "Field Reading"=1.2432314539284337e-05}, {0.0016840713634999997, "Field Reading"=1.2555545539639968e-05}, {0.0016784991494999998, "Field Reading"=1.2541091688057836e-05}, {0.0016910237845, "Field Reading"=1.263048584216377e-05}, {0.0016915083635, "Field Reading"=1.2797897502434403e-05}, {0.0016965419385000003, "Field Reading"=1.2726535846172536e-05}, {0.0017010910945000003, "Field Reading"=1.2745961009995105e-05}, {0.001703796989, "Field Reading"=1.2917956833801598e-05}, {0.00170688755, "Field Reading"=1.2917469303121321e-05}, {0.001707664419, "Field Reading"=1.2765067627113538e-05}, {0.0017119950964999998, "Field Reading"=1.2803390526632455e-05}, {0.0017115745155, "Field Reading"=1.2722823441897859e-05}, {0.0017213616355000003, "Field Reading"=1.2778583363926008e-05}, {0.0017282447114999998, "Field Reading"=1.3144947816597079e-05}, {0.0017284005130000003, "Field Reading"=1.3274440874788857e-05}, {0.001731701192, "Field Reading"=1.3210636544357726e-05}, {0.001742356883, "Field Reading"=1.3054043650462941e-05}, {0.0017433505900000003, "Field Reading"=1.3345643006104111e-05}, {0.0017431066895, "Field Reading"=1.3305779208668249e-05}, {0.001749731711, "Field Reading"=1.3139300138896654e-05}, {0.0017507466199999998, "Field Reading"=1.3117664548683963e-05}, {0.0017505856815000001, "Field Reading"=1.3403881674767984e-05}, {0.0017576411475000002, "Field Reading"=1.3295446203823522e-05}, {0.001761409849, "Field Reading"=1.3337679295251491e-05}, {0.0017673979494999999, "Field Reading"=1.3426647537802595e-05}, {0.0017730479269999998, "Field Reading"=1.3689473157779278e-05}, {0.0017789520075000003, "Field Reading"=1.3748443621066925e-05}, {0.0017824337755000003, "Field Reading"=1.3366937519552143e-05}, {0.0017856890155, "Field Reading"=1.3435929773205947e-05}, {0.001790526215, "Field Reading"=1.3436220728066282e-05}, {0.0017986648719999997, "Field Reading"=1.3559229288916855e-05}, {0.0017990182885, "Field Reading"=1.364010222967718e-05}, {0.0018040684229999999, "Field Reading"=1.3942800986999073e-05}, {0.001804471384, "Field Reading"=1.3443582455218259e-05}, {0.0018030768309999997, "Field Reading"=1.348402869549923e-05}, {0.0018051130485000001, "Field Reading"=1.3166505301922531e-05}, {0.0018123356160000003, "Field Reading"=1.3298094651893737e-05}, {0.0018098047425, "Field Reading"=1.313713454317292e-05}, {0.00181670879, "Field Reading"=1.3280828583388965e-05}, {0.0018216734294999998, "Field Reading"=1.2937585038712831e-05}, {0.0018228823949999998, "Field Reading"=1.3098421640461033e-05}, {0.0018323140005000002, "Field Reading"=1.3675083624963898e-05}, {0.0018358274219999998, "Field Reading"=1.3309173927582334e-05}, {0.0018364287345, "Field Reading"=1.3347185451700443e-05}, {0.001839584853, "Field Reading"=1.3154966039249278e-05}, {0.0018402510655000002, "Field Reading"=1.3336907241027693e-05}, {0.001846503147, "Field Reading"=1.3515846232641727e-05}, {0.0018495089835, "Field Reading"=1.3364380398580744e-05}, {0.0018614231275, "Field Reading"=1.3138382315377012e-05}, {0.0018652508359999996, "Field Reading"=1.3211882875238594e-05}, {0.0018650825200000002, "Field Reading"=1.3702979862180427e-05}, {0.0018674646824999998, "Field Reading"=1.3391920283383093e-05}, {0.001871475228, "Field Reading"=1.3435916088265104e-05}, {0.0018802515459999999, "Field Reading"=1.336818940575651e-05}, {0.001881180063, "Field Reading"=1.3256227050037881e-05}, {0.0018836065555, "Field Reading"=1.3153074891885698e-05}, {0.0018844740040000001, "Field Reading"=1.3344154394721994e-05}, {0.0018859175865, "Field Reading"=1.3232943228622393e-05}, {0.0018934621234999998, "Field Reading"=1.3086387587421383e-05}, {0.001901464857, "Field Reading"=1.331690938704351e-05}, {0.0019062248394999999, "Field Reading"=1.3014226992535158e-05}, {0.0019073106455, "Field Reading"=1.3148362591099246e-05}, {0.001912959958, "Field Reading"=1.3184692511896278e-05}, {0.0019177265200000001, "Field Reading"=1.3125415863298024e-05}, {0.001919319605, "Field Reading"=1.3224779859835617e-05}, {0.0019217171174999998, "Field Reading"=1.3154282461918645e-05}, {0.0019241282024999996, "Field Reading"=1.314867893944272e-05}, {0.0019249497935000005, "Field Reading"=1.312826569455102e-05}, {0.0019330273735, "Field Reading"=1.3114610218472158e-05}, {0.0019363632719999995, "Field Reading"=1.3164648761972917e-05}, {0.0019398894885000004, "Field Reading"=1.3113241974678131e-05}, {0.0019394641665, "Field Reading"=1.3337962229102173e-05}, {0.00194488622, "Field Reading"=1.3130068572415576e-05}, {0.0019511908710000002, "Field Reading"=1.3222557654366676e-05}, {0.0019525923654999996, "Field Reading"=1.3109329094935294e-05}, {0.0019519746429999998, "Field Reading"=1.3012879307920067e-05}, {0.0019550261445, "Field Reading"=1.3128654965519298e-05}, {0.0019608395485, "Field Reading"=1.3131279344149864e-05}, {0.0019673751175, "Field Reading"=1.3182781637326807e-05}, {0.0019721896985, "Field Reading"=1.3146981337926338e-05}, {0.0019770528135, "Field Reading"=1.3043543208902749e-05}, {0.001982117793, "Field Reading"=1.3025619920768175e-05}, {0.0019819501744999996, "Field Reading"=1.2973101371988902e-05}, {0.001980458725, "Field Reading"=1.2968738990371378e-05}, {0.0019878052475, "Field Reading"=1.2947781676783497e-05}, {0.001990118489, "Field Reading"=1.299616977022658e-05}, {0.0019943127415, "Field Reading"=1.2954916605354282e-05}, {0.0019997469729999997, "Field Reading"=1.2981650388071655e-05}, {0.0020045640335, "Field Reading"=1.2930133408121383e-05}, {0.002009950445, "Field Reading"=1.2971049561645105e-05}, {0.00201030414, "Field Reading"=1.31024886849717e-05}, {0.0020172990215, "Field Reading"=1.295373337346212e-05}, {0.002020535471, "Field Reading"=1.3028904429734091e-05}, {0.0020239874800000003, "Field Reading"=1.2894564223715039e-05}, {0.0020290527145, "Field Reading"=1.2956324592488754e-05}, {0.002031974369, "Field Reading"=1.2974730955846027e-05}, {0.0020346927375, "Field Reading"=1.2933963728203451e-05}, {0.0020363437094999995, "Field Reading"=1.2979699149874695e-05}, {0.00203733498, "Field Reading"=1.3011849084253809e-05}, {0.002045469146, "Field Reading"=1.2959220322049073e-05}, {0.0020469475640000003, "Field Reading"=1.291213134675763e-05}, {0.0020586598545000003, "Field Reading"=1.3070503828513883e-05}, {0.0020591374075, "Field Reading"=1.3011874471748771e-05}, {0.0020638504955, "Field Reading"=1.3046660257495448e-05}, {0.0020655298305, "Field Reading"=1.3095909952188556e-05}, {0.0020713746219999996, "Field Reading"=1.305764446468945e-05}, {0.0020697032040000005, "Field Reading"=1.3000483038881252e-05}, {0.0020765521285000003, "Field Reading"=1.2985576559541331e-05}, {0.0020774054379999996, "Field Reading"=1.3043810101690855e-05}, {0.0020806687339999996, "Field Reading"=1.3039941654248881e-05}, {0.0020862616440000003, "Field Reading"=1.2921526747197503e-05}, {0.002090200678, "Field Reading"=1.2921914050921462e-05}, {0.0020929801154999997, "Field Reading"=1.3006244891062116e-05}, {0.0020974899245, "Field Reading"=1.300127304018177e-05}, {0.0021008884824999996, "Field Reading"=1.2901231243312602e-05}, {0.0021037043225, "Field Reading"=1.2956886467050087e-05}, {0.0021115420425, "Field Reading"=1.2998052715809923e-05}, {0.0021187315395000002, "Field Reading"=1.297275726773137e-05}, {0.0021192939914999997, "Field Reading"=1.2969514583256798e-05}, {0.0021263486979999995, "Field Reading"=1.2911812064227905e-05}, {0.00212962384, "Field Reading"=1.2934915942311535e-05}, {0.0021315658395, "Field Reading"=1.2969461791935694e-05}, {0.0021323767519999997, "Field Reading"=1.2984194021945497e-05}, {0.0021412666285, "Field Reading"=1.3001385791267198e-05}, {0.0021423461285000004, "Field Reading"=1.305465983740958e-05}, {0.0021446447495, "Field Reading"=1.3052465232454396e-05}, {0.0021494816029999997, "Field Reading"=1.2952957774938617e-05}, {0.0021533983435, "Field Reading"=1.2897455058121717e-05}, {0.0021605384794999996, "Field Reading"=1.2968928254946945e-05}, {0.002164604849, "Field Reading"=1.3053392475054342e-05}, {0.0021672216520000004, "Field Reading"=1.297973825755906e-05}, {0.0021697240260000004, "Field Reading"=1.2975145592478813e-05}, {0.0021778564674999994, "Field Reading"=1.301479977980481e-05}, {0.0021806094504999997, "Field Reading"=1.2963775171722e-05}, {0.002187115433, "Field Reading"=1.2992512990159451e-05}, {0.0021936698759999996, "Field Reading"=1.2970490612575123e-05}, {0.0021904432690000005, "Field Reading"=1.3069430058684156e-05}, {0.0021968512780000003, "Field Reading"=1.3014803396728695e-05}, {0.002197999481, "Field Reading"=1.3046901042329241e-05}, {0.0022041311549999996, "Field Reading"=1.3040428399693919e-05}, {0.0022052790999999997, "Field Reading"=1.3118523442917656e-05}, {0.0022045199594999997, "Field Reading"=1.3047192032671192e-05}, {0.0022101015944999995, "Field Reading"=1.3046461656205289e-05}, {0.0022153682449999996, "Field Reading"=1.310033147595164e-05}, {0.0022195349759999996, "Field Reading"=1.3056778233218226e-05}, {0.002225388589, "Field Reading"=1.3062695147547402e-05}, {0.002229183916, "Field Reading"=1.3064579929091838e-05}, {0.0022313903034999996, "Field Reading"=1.3046228960106534e-05}, {0.0022355979184999998, "Field Reading"=1.3094846830633943e-05}, {0.0022436847835, "Field Reading"=1.3107060845814117e-05}, {0.0022426261764999997, "Field Reading"=1.3103371099071528e-05}, {0.0022446627769999996, "Field Reading"=1.3077630868929654e-05}, {0.002247795897, "Field Reading"=1.3180536391710655e-05}, {0.0022554874755, "Field Reading"=1.3127475759896741e-05}, {0.002251914621, "Field Reading"=1.3113888184937383e-05}, {0.002254543202, "Field Reading"=1.3086561175964867e-05}, {0.0022582395355000002, "Field Reading"=1.3122047467297258e-05}, {0.002262866221, "Field Reading"=1.3101977099035917e-05}, {0.0022632819854999995, "Field Reading"=1.3098236626453223e-05}, {0.0022661053169999996, "Field Reading"=1.3118871969818777e-05}, {0.0022719533974999992, "Field Reading"=1.3148112904442982e-05}, {0.002280884177, "Field Reading"=1.3162681141895323e-05}, {0.0022845083755, "Field Reading"=1.3156055162756559e-05}, {0.0022898250915, "Field Reading"=1.316675727812337e-05}, {0.0022930354460000005, "Field Reading"=1.3191476285407504e-05}, {0.002297341805, "Field Reading"=1.3208765145536307e-05}, {0.0023021415015, "Field Reading"=1.3209813996052508e-05}, {0.0023075912340000003, "Field Reading"=1.3171420914837744e-05}, {0.002311992324, "Field Reading"=1.3206617472310487e-05}, {0.0023175748774999995, "Field Reading"=1.324952784855145e-05}, {0.0023228883435000005, "Field Reading"=1.3214600620036088e-05}, {0.0023248942600000004, "Field Reading"=1.3249441732465759e-05}, {0.0023306576069999996, "Field Reading"=1.3278635010704024e-05}, {0.002328151921, "Field Reading"=1.3217098953924467e-05}, {0.0023319565095, "Field Reading"=1.3204855645504154e-05}, {0.0023346804929999998, "Field Reading"=1.3249504833053795e-05}, {0.0023355887054999996, "Field Reading"=1.331259989674859e-05}, {0.0023323139870000003, "Field Reading"=1.3250306380685435e-05}, {0.0023362469065, "Field Reading"=1.3233401918481398e-05}, {0.0023389747485000004, "Field Reading"=1.3236704480630724e-05}, {0.0023437284970000004, "Field Reading"=1.3199452107183353e-05}, {0.0023486378595000005, "Field Reading"=1.3260219219203588e-05}, {0.002353789604, "Field Reading"=1.3233607721820609e-05}, {0.0023548495035000004, "Field Reading"=1.326019356746296e-05}, {0.0023550155599999997, "Field Reading"=1.3264600495897255e-05}, {0.0023600299665000003, "Field Reading"=1.3275528368691777e-05}, {0.002357892157, "Field Reading"=1.3236423037667356e-05}, {0.0023630866944999995, "Field Reading"=1.3295251219317754e-05}, {0.0023682346440000003, "Field Reading"=1.3257389534232334e-05}, {0.0023699970134999997, "Field Reading"=1.3321121714643843e-05}, {0.0023746077175, "Field Reading"=1.331029580418595e-05}, {0.002380768248, "Field Reading"=1.3301661776088048e-05}, {0.002382166243, "Field Reading"=1.3334622679232035e-05}, {0.002386489845, "Field Reading"=1.326113842459557e-05}, {0.0023854349114999997, "Field Reading"=1.3296900731685586e-05}, {0.0023892443405, "Field Reading"=1.3260097573234767e-05}, {0.0023905629235, "Field Reading"=1.3281134678957457e-05}, {0.0023946556585, "Field Reading"=1.3207770371309443e-05}, {0.002395663622, "Field Reading"=1.3221040130985402e-05}, {0.0024020718085000004, "Field Reading"=1.3272720848115725e-05}, {0.0024038628114999997, "Field Reading"=1.3182660260974909e-05}, {0.0024092676249999998, "Field Reading"=1.3200881539550086e-05}, {0.0024101021064999997, "Field Reading"=1.3230761545484155e-05}, {0.002412250205, "Field Reading"=1.3259260364062309e-05}, {0.00241070687, "Field Reading"=1.3197603817248233e-05}, {0.0024157253750000003, "Field Reading"=1.327979697308101e-05}, {0.002419046429499999, "Field Reading"=1.3286256907067119e-05}, {0.0024193681770000005, "Field Reading"=1.328565490963133e-05}, {0.0024288468084999997, "Field Reading"=1.3182889845235993e-05}, {0.0024357376114999994, "Field Reading"=1.3195690059568667e-05}]
  out "data":dbl[](array[numeric])=[-9.479e-06, 17491.89, 0.0024357376114999994, 3.066255043659346e-10, 2.3236791935984393e-05, 1.3195690059568667e-05, -1.5999999999999879, -7.999999999999939e-08]
  in  "Nanovoltmeter 2182a VISA":refnum<visa-resource-name>="GPIB0::4::INSTR"
  in  "Step":dbl[](array[numeric])=[0.005, 0.001, 0.005] min=-3000.0 max=3000.0 format="%.1e"
  in  "To":dbl[](array[numeric])=[0.36, -0.06, -1.6] min=-3000.0 max=3000.0 format="%.1e"
  in  "From":dbl[](array[numeric])=[1.6, 0.36, -0.06] min=-3000.0 max=3000.0 format="%.1e"
  in  "file name":string="027_MA2087_STS_[Dev100]_baseT_1T_measureR_40uV_137.919Hz_float_100xaverage"
  out "File path":path=path "D:/Pranava/Data/STS/MA2087/026_MA2087_STS_[Dev100]_baseT_0T_measureR_40uV_137.919Hz_float_100xaverage.dat"
  # ".dat"
  # "Set Voltage (V)"
  # "Set Magnetic Field (T)"
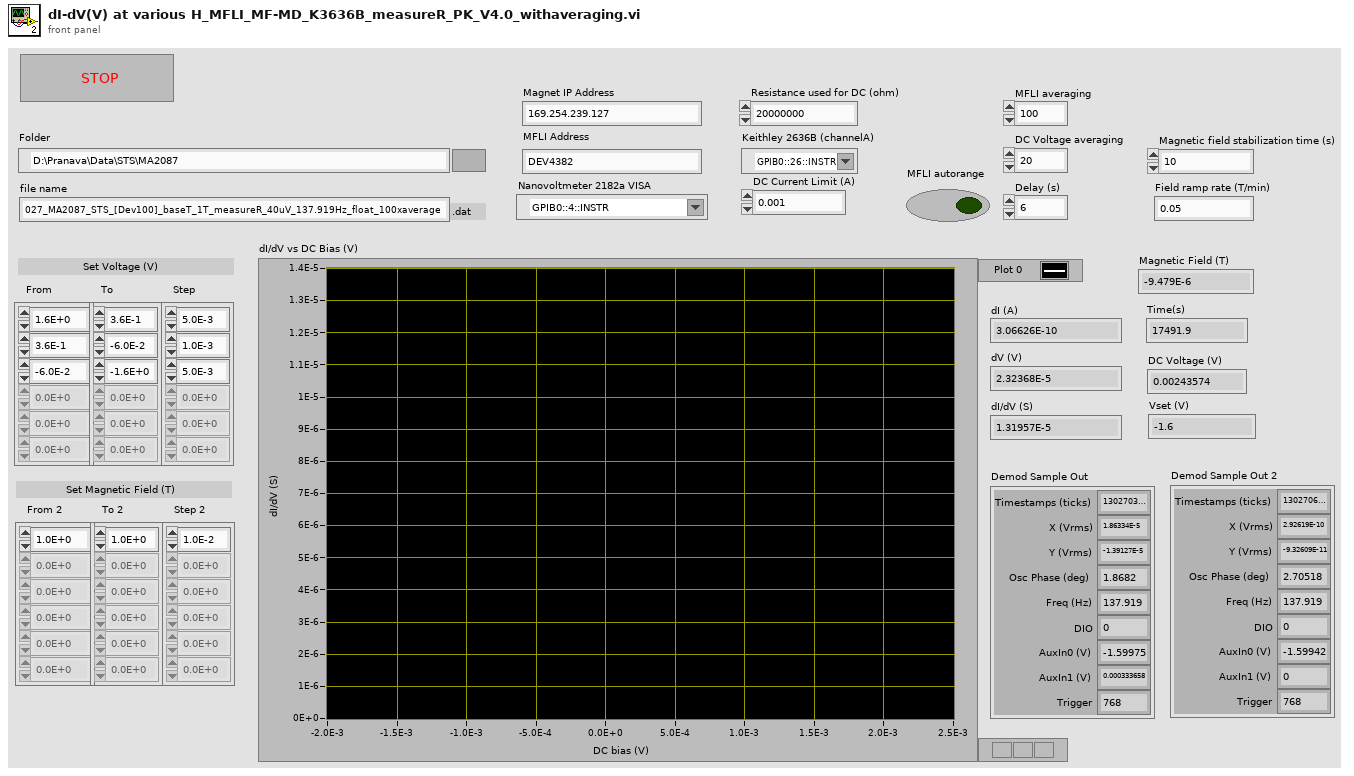
[diagram p1: front panel]
types:
  T1 = typedef "Zurich Instruments LabOne.lvlib/ziTypeDemodSampleSingle.ctl" = cluster{"Timestamps (ticks)":u64, "X (Vrms)":dbl, "Y (Vrms)":dbl, "Osc Phase (deg)":dbl, "Freq (Hz)":dbl, "DIO":u32, "AuxIn0 (V)":dbl, "AuxIn1 (V)":dbl, "Trigger":u32}
  T2 = enum16{"open", "replace", "create", "open or create", "replace or create", "replace or create with confirmation"}
  T3 = typedef "Zurich Instruments LabOne.lvlib/ziTypeHandle.ctl" = cluster{"handleValid":bool, "Conn":u64, "Path Prefix":string, "Handle":u64, "Connected":bool, "Clockbase(s)":dbl}
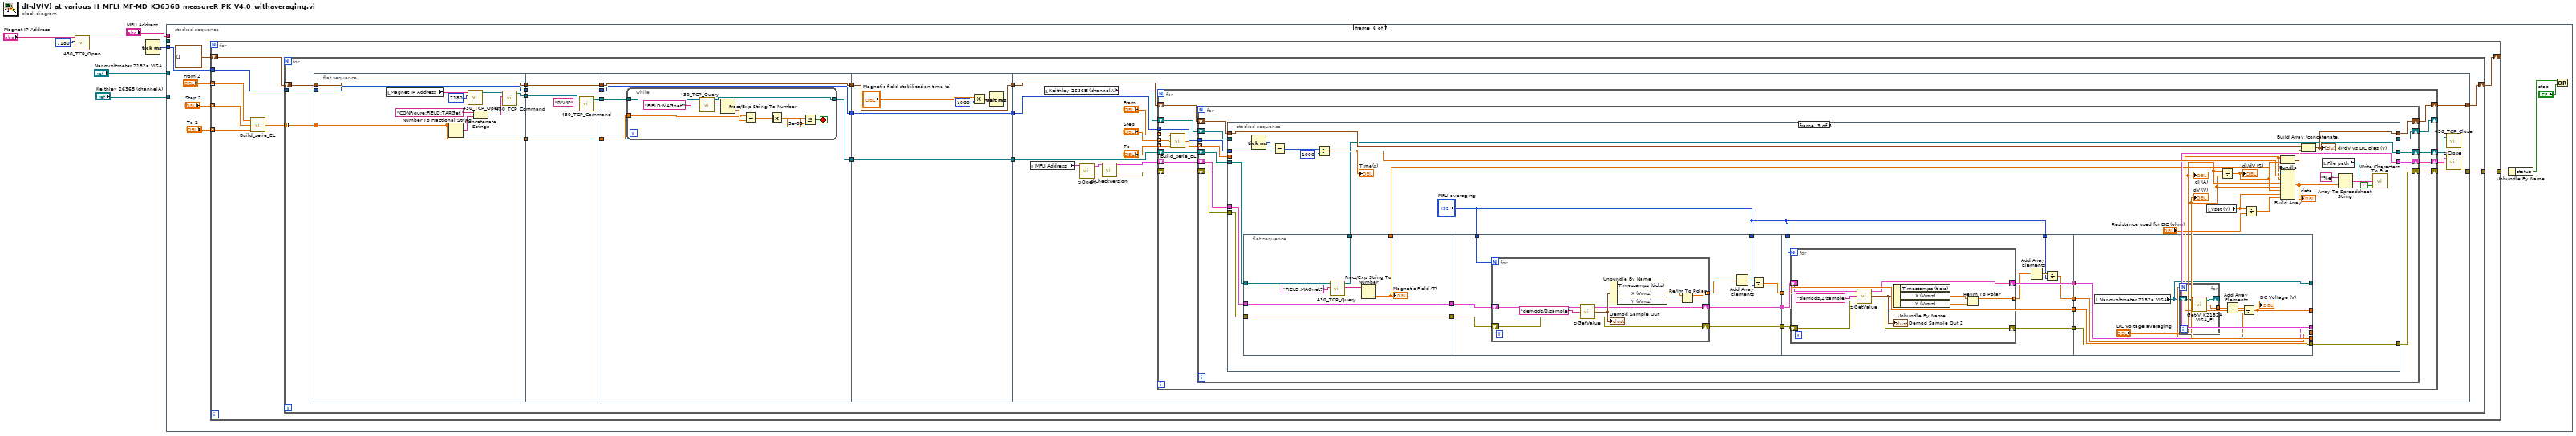
[diagram p0: block diagram]
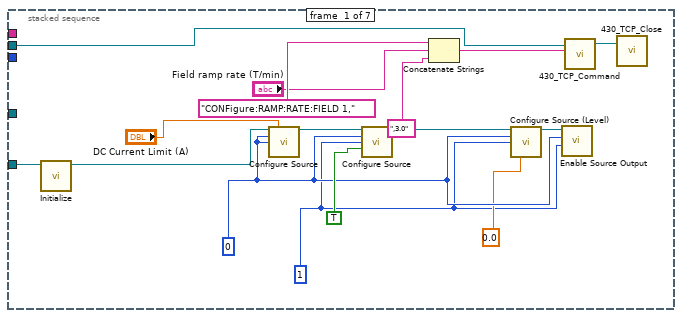
[diagram p2: hidden frame]
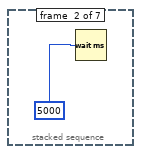
[diagram p3: hidden frame]
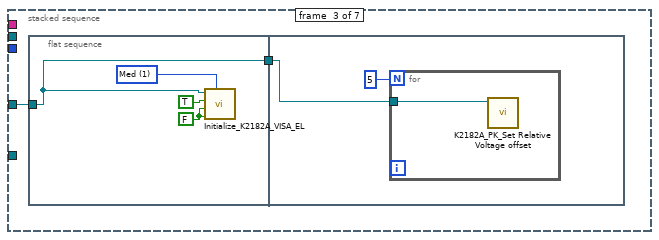
[diagram p4: hidden frame]
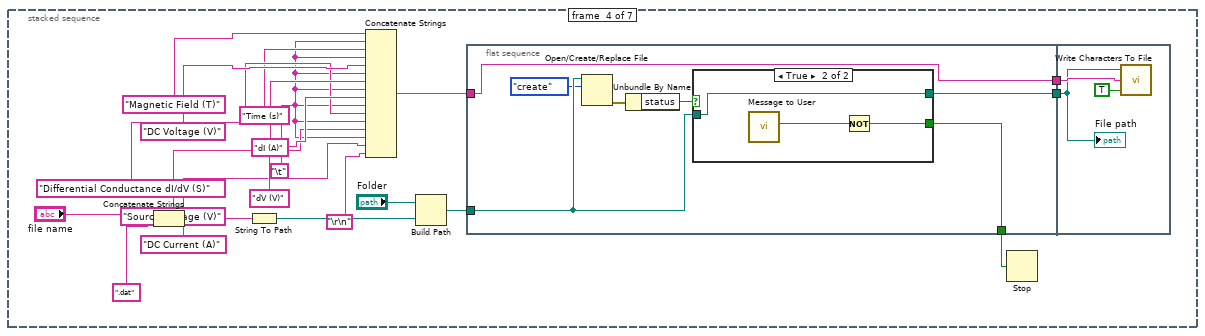
[diagram p5: hidden frame]
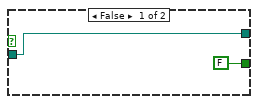
[diagram p6: hidden frame]
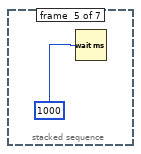
[diagram p7: hidden frame]
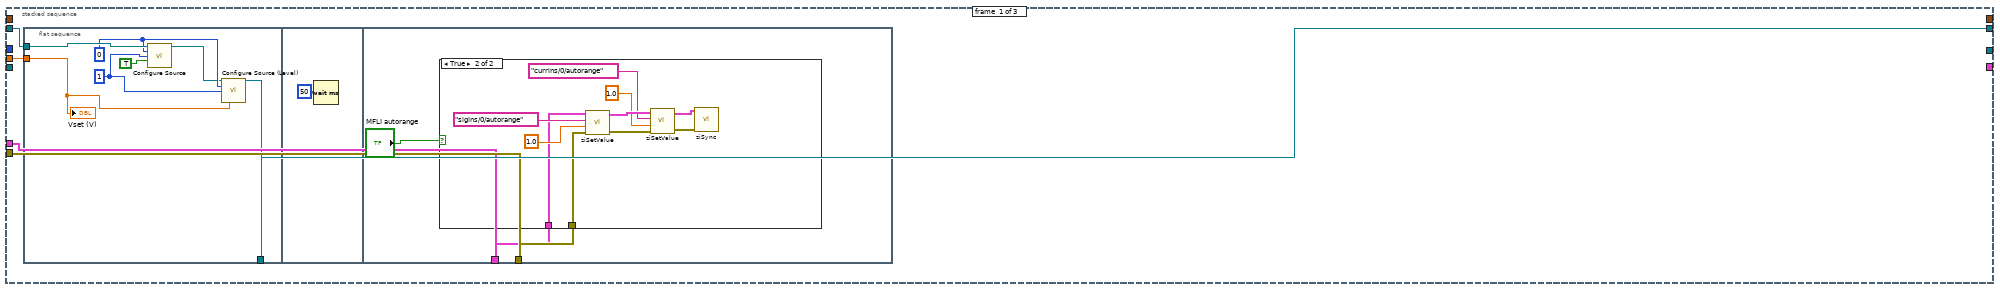
[diagram p8: hidden frame]
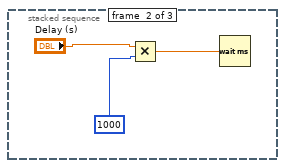
[diagram p10: hidden frame]
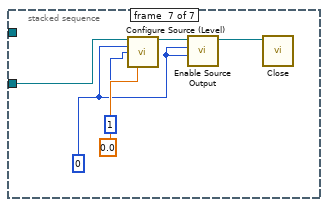
[diagram p11: hidden frame]
diagram:
  n1 = call "430_TCP_Open.vi"("IP Address"="Magnet IP Address", "TCP Port"=7180) -> ("connection ID"=w2:refnum<k5>)  [unwired: 4 in, 2 out]
  n2 = Tick Count (ms)() -> (millisecond timer value=w5:u32)
  n3 = stacked-sequence {
    tunnel: "Nanovoltmeter 2182a VISA" -> [_ _ w26 _ _ _ _]
    tunnel: "MFLI Address" -> [_ _ _ _ _ _ _]
    tunnel: w5 -> [_ _ _ _ _ w76 _]
    tunnel: w2 -> [w18 _ _ _ _ _ _]
    tunnel: "Keithley 2636B (channelA)" -> [w17 _ _ _ _ _ w309]
    frame #0 {
      w11 = 0
      w8 = 1
      n4 = call <instrlib>:"Initialize.vi"("VISA resource name"=w17) -> ("VISA resource name out"=w16:refnum<visa-resource-name>)  [unwired: 9 in, 1 out]
      n5 = call-poly <instrlib>:"Configure Source.vi"("VISA resource name"=w16, "Current Limit (0.1 A)"="DC Current Limit (A)", "Source Measure Unit Channel (0: Channel A)"=w11, "Limit Type (1: Voltage)"=w11) -> ("VISA resource name out"=w15:refnum<visa-resource-name>)  [unwired: 10 in, 1 out]
      n6 = call-poly <instrlib>:"Configure Source.vi"("VISA resource name"=w15, "Source Measure Unit Channel (0: Channel A)"=w11, "Range Type (1: Voltage)"=w8, "Auto Range (T: Enable)"=TRUE) -> ("VISA resource name out"=w14:refnum<visa-resource-name>)  [unwired: 10 in, 1 out]
      n7 = Concatenate Strings("CONFigure:RAMP:RATE:FIELD 1," ("String"), "Field ramp rate (T/min)", ",3.0") -> (w19:string)
      n8 = call <instrlib>:"Configure Source (Level).vi"("VISA resource name"=w14, "Source Measure Unit Channel (0: Channel A)"=w11, "Level Type (1: Voltage)"=w8, "Voltage Level (0 V)"=0.0) -> ("VISA resource name out"=w13:refnum<visa-resource-name>)  [unwired: 10 in, 1 out]
      n9 = call <instrlib>:"Enable Source Output.vi"("Output Mode (0: Turn off)"=w8, "Source Measure Unit Channel (0: Channel A)"=w11, "VISA resource name"=w13) -> ()  [unwired: 7 in, 2 out]
      n10 = call "430_TCP_Command.vi"("Command"=w19, "connection ID"=w18) -> ("connection ID out"=w23:refnum<k5>)  [unwired: 2 in, 2 out]
      n11 = call "430_TCP_Close.vi"("connection ID"=w23) -> ()  [unwired: 1 in, 2 out]
    }
    frame #1 {
      n12 = Wait (ms)(milliseconds to wait=5000) -> ()  [unwired: 1 out]
    }
    frame #2 {
      n13 = flat-sequence {
        tunnel: w26 -> [w27]
        tunnel: [w27] -> w25
        tunnel: w25 -> [w31]
        frame #0 {
          w29 = u16 1 items=["Slow", "Med", "Fast"] ("Rate (NPLC)")
          w30 = FALSE ("Auto range?")
          n14 = call "Initialize_K2182A_VISA_EL.vi"("VISA address"=w27, "Auto range?"=TRUE, "Analog LPass\nFilter?"=w30, "DC\nFilter?"=w30, "Rate (NPLC)"=w29) -> ()  [unwired: 2 in]
        }
        frame #1 {
          n15 = for {
            N: 5 ("Numeric") -> [_]
            tunnel: w31 -> [w33]
            n16 = call "K2182A_PK_Set Relative Voltage offset.vi"("VISA address"=w33) -> ()  [unwired: 11 in]
          }
        }
      }
    }
    frame #3 {
      w35 = "\t"
      n17 = Concatenate Strings("file name", ".dat" ("string")) -> (w50:string)
      n18 = String To Path(string=w50) -> (path=w42:path)
      n19 = Concatenate Strings("Magnetic Field (T)", w35, "Time (s)", w35, "DC Voltage (V)" ("string"), w35, "dI (A)" ("string"), w35, "dV (V)" ("string"), w35, "Differential Conductance dI/dV (S)", w35, "Source Voltage (V)", w35, "DC Current (A)", "\r\n") -> (w51:string)
      n20 = Build Path(base path="Folder", name or relative path=w42) -> (appended path=w41:path)
      n21 = flat-sequence {
        tunnel: w41 -> [w57]
        tunnel: w51 -> [w60]
        tunnel: [w60] -> w53
        tunnel: [w59] -> w48
        tunnel: [w58] -> w52
        tunnel: w53 -> [w67]
        tunnel: w52 -> [w66]
        frame #0 {
          n22 = Open/Create/Replace File(file path (use dialog)=w57, operation (0:open)=T2."create") -> (error out=w56:errorcluster)  [unwired: 4 in, 2 out]
          n23 = Unbundle By Name(w56) -> ("status"=w54:bool)
          n24 = case shown="True" w54 {
            tunnel: [FALSE ("Yes") w64] -> w59
            tunnel: [w61 w63] -> w58
            tunnel: w57 -> [w61 w63]
            frame False {
            }
            frame True {
              n25 = call "Message to User"() -> ("Yes"=w65:bool)  [unwired: 10 in, 1 out]
              n26 = Not(x=w65) -> (.not. x?=w64:bool)
            }
          }
        }
        frame #1 {
          n27 = call <vilib>:"Write Characters To File.vi"("append to file? (new file:F)"=TRUE, "character string"=w67, "file path (dialog if empty)"=w66) -> ()  [unwired: 2 in, 1 out]
          "File path" <- w66
        }
      }
      n28 = Stop(stop? (T)=w48) -> ()
    }
    frame #4 {
      n29 = Wait (ms)(milliseconds to wait=u32 1000) -> ()  [unwired: 1 out]
    }
    frame #5 {
      n30 = for {
        tunnel: w76 -> [w84]
        tunnel: "From 2" -> [w83] mode=indexing
        tunnel: "Step 2" -> [w82] mode=indexing
        tunnel: "To 2" -> [w81] mode=indexing
        shift-right: [w80] -> _
        shift-left: cluster{dbl, "Field Reading":dbl}[] [] -> [w85]
        tunnel: [w78] -> w71
        n31 = call "Build_serie_EL.vi"("end value"=w81, "increment"=w82, "start value"=w83) -> ("output array"=w79:dbl[])
        n32 = for {
          tunnel: w84 -> [w95]
          shift-right: [w94] -> w80
          shift-left: w85 -> [w96]
          tunnel: w79 -> [w93] mode=indexing
          tunnel: [w86] -> w78
          n33 = flat-sequence {
            tunnel: w95 -> [w113]
            tunnel: w96 -> [w114]
            tunnel: [w114] -> w104
            tunnel: [w113] -> w103
            tunnel: w93 -> [w105]
            tunnel: [w106] -> w92
            tunnel: [w105] -> w89
            tunnel: [w120] -> w102
            tunnel: [w119] -> w101
            tunnel: w104 -> [w120]
            tunnel: w103 -> [w119]
            tunnel: w92 -> [w117]
            tunnel: [w116] -> w91
            tunnel: [w115] -> w90
            tunnel: w89 -> [w115]
            tunnel: [w125] -> w100
            tunnel: [w124] -> w99
            tunnel: w102 -> [w125]
            tunnel: w101 -> [w124]
            tunnel: w91 -> [w123]
            tunnel: w90 -> [w122]
            tunnel: [w121] -> w87
            tunnel: [w141] -> w98
            tunnel: [w140] -> w97
            tunnel: w100 -> [w141]
            tunnel: w99 -> [w140]
            tunnel: [w136] -> w88
            tunnel: w87 -> [w136]
            tunnel: [w152] -> w86
            tunnel: w98 -> [w154]
            tunnel: w97 -> [w153]
            tunnel: [w151] -> w94
            tunnel: w88 -> [w150]
            frame #0 {
              n34 = local read "Magnet IP Address"() -> (w108:string)
              n35 = Number To Fractional String(number=w105) -> (F-format string=w110:string)  [unwired: 3 in]
              n36 = call "430_TCP_Open.vi"("IP Address"=w108, "TCP Port"=7180) -> ("connection ID"=w107:refnum<k5>)  [unwired: 4 in, 2 out]
              n37 = Concatenate Strings("CONFigure:FIELD:TARGet " ("String"), w110) -> (w112:string)
              n38 = call "430_TCP_Command.vi"("Command"=w112, "connection ID"=w107) -> ("connection ID out"=w106:refnum<k5>)  [unwired: 2 in, 2 out]
            }
            frame #1 {
              n39 = call "430_TCP_Command.vi"("Command"="RAMP", "connection ID"=w117) -> ("connection ID out"=w116:refnum<k5>)  [unwired: 2 in, 2 out]
            }
            frame #2 {
              n40 = while {
                tunnel: w123 -> [w135]
                tunnel: w122 -> [w130]
                tunnel: [w126] -> w121
                stop <- w128 stop-if-true
                n41 = call "430_TCP_Query.vi"("Command"="FIELD:MAGnet?" ("String"), "connection ID"=w135) -> ("Response"=w134:string, "connection ID out"=w126:refnum<k5>)  [unwired: 5 in, 3 out]
                n42 = Fract/Exp String To Number(string=w134) -> (number=w131:dbl)  [unwired: 3 in, 1 out]
                n43 = Subtract(x=w130, y=w131) -> (x-y=w133:dbl)
                n44 = Absolute Value(x=w133) -> (abs(x)=w132:dbl)
                n45 = Less Or Equal?(x=w132, y=5e-05) -> (x <= y?=w128:bool)
              }
            }
            frame #3 {
              n46 = Multiply(x="Magnetic field stabilization time (s)", y=1000) -> (x*y=w138:dbl)
              n47 = Wait (ms)(milliseconds to wait=w138) -> ()  [unwired: 1 out]
            }
            frame #4 {
              n48 = local read "MFLI Address"() -> (w147:string)
              n49 = local read "Keithley 2636B (channelA)"() -> (w142:refnum<visa-resource-name>)
              n50 = call <instrlib>:"ziOpen.vi"("Address"=w147) -> ("Error Out"=w146:errorcluster, "HandleOut"=w149:T3)  [unwired: 3 in, 1 out]
              n51 = call <instrlib>:"ziCheckVersion.vi"("Handle In"=w149, "Error In"=w146) -> ("Handle Out"=w148:T3, "Error Out"=w145:errorcluster)  [unwired: 11 in, 1 out]
              n52 = for {
                tunnel: "From" -> [w169] mode=indexing
                tunnel: "To" -> [w168] mode=indexing
                tunnel: "Step" -> [w167] mode=indexing
                shift-right: [w171] -> w151
                shift-left: w154 -> [w172]
                tunnel: w153 -> [w166]
                shift-right: [w164] -> w144
                shift-left: w148 -> [w165]
                shift-right: [w163] -> w152
                shift-left: w145 -> [w162]
                shift-right: [w160] -> w143
                shift-left: w150 -> [w161]
                shift-right: [w158] -> _
                shift-left: w142 -> [w159]
                n53 = call "Build_serie_EL.vi"("end value"=w168, "increment"=w167, "start value"=w169) -> ("output array"=w170:dbl[])
                n54 = for {
                  tunnel: w170 -> [w184] mode=indexing
                  shift-right: [w182] -> w171
                  shift-left: w172 -> [w183]
                  tunnel: w166 -> [w181]
                  shift-right: [w179] -> w164
                  shift-left: w165 -> [w180]
                  shift-right: [w178] -> w163
                  shift-left: w162 -> [w177]
                  shift-right: [w175] -> w160
                  shift-left: w161 -> [w176]
                  shift-right: [w173] -> w158
                  shift-left: w159 -> [w174]
                  n55 = stacked-sequence {
                    tunnel: w183 -> [_ _ w249]
                    tunnel: w184 -> [w189 _ _]
                    tunnel: [_ _ w248] -> w182
                    tunnel: w181 -> [_ _ w245]
                    tunnel: w180 -> [w185 _ w241]
                    tunnel: [_ _ w240] -> w179
                    tunnel: [_ _ w239] -> w178
                    tunnel: w177 -> [w186 _ w238]
                    tunnel: w176 -> [_ _ w223]
                    tunnel: [_ _ w222] -> w175
                    tunnel: w174 -> [w187 _ _]
                    tunnel: [w188 _ _] -> w173
                    frame #0 {
                      n56 = flat-sequence {
                        tunnel: w189 -> [w196]
                        tunnel: [w195] -> w188
                        tunnel: w187 -> [w194]
                        tunnel: w186 -> [w200]
                        tunnel: w185 -> [w199]
                        frame #0 {
                          w193 = 0
                          w192 = 1
                          n57 = call-poly <instrlib>:"Configure Source.vi"("VISA resource name"=w194, "Source Measure Unit Channel (0: Channel A)"=w193, "Range Type (1: Voltage)"=w192, "Auto Range (T: Enable)"=TRUE) -> ("VISA resource name out"=w190:refnum<visa-resource-name>)  [unwired: 10 in, 1 out]
                          n58 = call <instrlib>:"Configure Source (Level).vi"("VISA resource name"=w190, "Source Measure Unit Channel (0: Channel A)"=w193, "Level Type (1: Voltage)"=w192, "Voltage Level (0 V)"=w196) -> ("VISA resource name out"=w195:refnum<visa-resource-name>)  [unwired: 10 in, 1 out]
                          "Vset (V)" <- w196
                        }
                        frame #1 {
                          n59 = Wait (ms)(milliseconds to wait=50) -> ()  [unwired: 1 out]
                        }
                        frame #2 {
                          n60 = case shown="True" "MFLI autorange" {
                            tunnel: w200 -> [_ w202]
                            tunnel: w199 -> [_ w201]
                            frame False {
                            }
                            frame True {
                              n61 = call-poly <instrlib>:"ziSetValue.vi"("Error In"=w202, "Value"=1.0, "Path"="sigins/0/autorange", "Handle In"=w201) -> ("Error Out"=w208:errorcluster, "Handle Out"=w207:T3)  [unwired: 1 in]
                              n62 = call-poly <instrlib>:"ziSetValue.vi"("Error In"=w208, "Value"=1.0, "Path"="currins/0/autorange", "Handle In"=w207) -> ("Error Out"=w210:errorcluster, "Handle Out"=w209:T3)  [unwired: 1 in]
                              n63 = call <instrlib>:"ziSync.vi"("Handle In"=w209, "Error In"=w210) -> ()  [unwired: 12 in, 2 out]
                            }
                          }
                        }
                      }
                    }
                    frame #1 {
                      n64 = Multiply(x="Delay (s)", y=1000) -> (x*y=w212:dbl)
                      n65 = Wait (ms)(milliseconds to wait=w212) -> ()  [unwired: 1 out]
                    }
                    frame #2 {
                      n66 = flat-sequence {
                        tunnel: w238 -> [w256]
                        tunnel: w241 -> [w257]
                        tunnel: [w257] -> w225
                        tunnel: [w256] -> w224
                        tunnel: w223 -> [w253]
                        tunnel: [w252] -> w222
                        tunnel: [w251] -> w221
                        tunnel: [w264] -> w232
                        tunnel: [w263] -> w231
                        tunnel: [w260] -> w230
                        tunnel: w225 -> [w266]
                        tunnel: w224 -> [w265]
                        tunnel: "MFLI averaging" -> [w259]
                        tunnel: "MFLI averaging" -> [w258]
                        tunnel: w232 -> [w285]
                        tunnel: w231 -> [w284]
                        tunnel: w230 -> [w281]
                        tunnel: [w283] -> w229
                        tunnel: [w282] -> w228
                        tunnel: [w279] -> w227
                        tunnel: [w281] -> w226
                        tunnel: "MFLI averaging" -> [w277]
                        tunnel: "MFLI averaging" -> [w276]
                        tunnel: [w300] -> w217
                        tunnel: [w301] -> w218
                        tunnel: [w302] -> w239
                        tunnel: [w303] -> w240
                        tunnel: w229 -> [w303]
                        tunnel: w228 -> [w302]
                        tunnel: w227 -> [w301]
                        tunnel: w226 -> [w300]
                        tunnel: [w297] -> w216
                        tunnel: [w295] -> _
                        frame #0 {
                          n67 = call "430_TCP_Query.vi"("Command"="FIELD:MAGnet?" ("String"), "connection ID"=w253) -> ("Response"=w255:string, "connection ID out"=w252:refnum<k5>)  [unwired: 5 in, 3 out]
                          n68 = Fract/Exp String To Number(string=w255) -> (number=w251:dbl)  [unwired: 3 in, 1 out]
                          "Magnetic Field (T)" <- w251
                        }
                        frame #1 {
                          n69 = for {
                            N: w258 -> [_]
                            tunnel: [w269] -> w261 mode=indexing
                            shift-right: [w271] -> w264
                            shift-left: w266 -> [w273]
                            shift-right: [w270] -> w263
                            shift-left: w265 -> [w272]
                            n70 = call-poly <instrlib>:"ziGetValue.vi"("error in"=w272, "Path"="demods/0/sample", "Handle In"=w273) -> ("error out"=w270:errorcluster, "Demod Sample Out"=w274:T1, "Handle Out"=w271:T3)
                            "Demod Sample Out" <- w274
                            n71 = Unbundle By Name(w274) -> ("X (Vrms)"=w268:dbl, "Y (Vrms)"=w267:dbl)  [unwired: 1 out]
                            n72 = Re/Im To Polar(2:w267, 3:w268) -> (1:w269:dbl)  [unwired: 1 out]
                          }
                          n73 = Add Array Elements(numeric array=w261) -> (sum=w262:dbl)
                          n74 = Divide(x=w262, y=w259) -> (x/y=w260:dbl)
                        }
                        frame #2 {
                          n75 = for {
                            N: w276 -> [_]
                            tunnel: [w286] -> w278 mode=indexing
                            shift-right: [w290] -> w283
                            shift-left: w285 -> [w292]
                            shift-right: [w289] -> w282
                            shift-left: w284 -> [w291]
                            n76 = call-poly <instrlib>:"ziGetValue.vi"("error in"=w291, "Path"="demods/2/sample", "Handle In"=w292) -> ("error out"=w289:errorcluster, "Demod Sample Out"=w293:T1, "Handle Out"=w290:T3)
                            "Demod Sample Out 2" <- w293
                            n77 = Unbundle By Name(w293) -> ("X (Vrms)"=w288:dbl, "Y (Vrms)"=w287:dbl)  [unwired: 1 out]
                            n78 = Re/Im To Polar(2:w287, 3:w288) -> (1:w286:dbl)  [unwired: 1 out]
                          }
                          n79 = Add Array Elements(numeric array=w278) -> (sum=w280:dbl)
                          n80 = Divide(x=w280, y=w277) -> (x/y=w279:dbl)
                        }
                        frame #3 {
                          n81 = local read "Nanovoltmeter 2182a VISA"() -> (w295:refnum<visa-resource-name>)
                          n82 = for {
                            N: "DC Voltage averaging" -> [_]
                            tunnel: [w305] -> w298 mode=indexing
                            shift-right: [w304] -> _
                            shift-left: w295 -> [w306]
                            n83 = call "Get-V_K2182A_VISA_EL.vi"("VISA K2182A"=w306) -> ("V (V)"=w305:dbl, "VISA K2182A"=w304:refnum<visa-resource-name>)  [unwired: 2 in, 1 out]
                          }
                          n84 = Add Array Elements(numeric array=w298) -> (sum=w299:dbl)
                          n85 = Divide(x=w299, y="DC Voltage averaging") -> (x/y=w297:dbl)
                          "DC Voltage (V)" <- w297
                        }
                      }
                      n86 = Tick Count (ms)() -> (millisecond timer value=w246:u32)
                      n87 = Subtract(x=w246, y=w245) -> (x-y=w244:u32)
                      n88 = Divide(x=w244, y=1000) -> (x/y=w242:dbl)
                      "Time(s)" <- w242
                      n89 = local read "Vset (V)"() -> (w219:dbl)
                      n90 = Divide(x=w218, y=w217) -> (x/y=w247:dbl)
                      "dI/dV (S)" <- w247
                      n91 = Divide(x=w219, y="Resistance used for DC (ohm)") -> (x/y=w215:dbl)
                      n92 = Bundle(w216, w247) -> (w250:cluster{dbl, dbl})  [unwired: 1 in]
                      n93 = Build Array(w221, w242, w216, w218, w217, w247, w219, w215) -> (w233:dbl[])
                      "data" <- w233
                      n94 = Build Array (concatenate)(w249, w250) -> (w248:cluster{dbl, "Field Reading":dbl}[])
                      "dI/dV vs DC Bias (V)" <- w248
                      n95 = local read "File path"() -> (w235:path)
                      n96 = Array To Spreadsheet String(array=w233, 3:"%e" ("format string")) -> (spreadsheet string=w236:string)  [unwired: 1 in]
                      n97 = call <vilib>:"Write Characters To File.vi"("append to file? (new file:F)"=TRUE, "character string"=w236, "file path (dialog if empty)"=w235) -> ()  [unwired: 2 in, 1 out]
                      "dI (A)" <- w218
                      "dV (V)" <- w217
                    }
                  }
                }
              }
              n98 = call "430_TCP_Close.vi"("connection ID"=w143) -> ()  [unwired: 1 in, 2 out]
              n99 = call <instrlib>:"ziClose.vi"("Handle In"=w144) -> ()  [unwired: 1 in, 4 out]
            }
          }
        }
      }
      n100 = Unbundle By Name(w71) -> ("status"=w70:bool)
      n101 = Or(x=w70, y="stop") -> ()  [unwired: 1 out]
    }
    frame #6 {
      w308 = 0
      n102 = call <instrlib>:"Configure Source (Level).vi"("VISA resource name"=w309, "Source Measure Unit Channel (0: Channel A)"=w308, "Level Type (1: Voltage)"=1, "Voltage Level (0 V)"=0.0) -> ("VISA resource name out"=w312:refnum<visa-resource-name>)  [unwired: 10 in, 1 out]
      n103 = call <instrlib>:"Enable Source Output.vi"("Output Mode (0: Turn off)"=w308, "Source Measure Unit Channel (0: Channel A)"=w308, "VISA resource name"=w312) -> ("VISA resource name out"=w307:refnum<visa-resource-name>)  [unwired: 7 in, 1 out]
      n104 = call <instrlib>:"Close.vi"("VISA resource name"=w307) -> ()  [unwired: 10 in, 1 out]
    }
  }
